vi "CIPT_softwarecontrol probe rework 8 8 23.vi"() -> ()   [LabVIEW 2022 SP3]
uses:
  Git/CIPT/CIPT/Labview Project/CIPT modes.ctl
  <vilib>/Analysis/baseanly.llb/Mean (DBL).vi
  <vilib>/Utility/file.llb/Read Delimited Spreadsheet (DBL).vi
  <vilib>/Utility/file.llb/Read Delimited Spreadsheet (I64).vi
  <vilib>/gmath/NumericalOptimization/Nonlinear Curve Fit LM.vi
  <vilib>/Utility/file.llb/Write Delimited Spreadsheet (string).vi
  <vilib>/Utility/file.llb/Write Delimited Spreadsheet (I64).vi
  <vilib>/Utility/file.llb/Write Delimited Spreadsheet (DBL).vi
  C:/CIPT/Labview Project/Camera Driver/Labview Driver/OtherDrivers/LabVIEW/ueye.NET/uEyeDotNet.dll
  CIPT/Labview Project/Camera Driver/Labview Driver/OtherDrivers/LabVIEW/ueye.NET/uEyeDotNet.dll
  <vilib>/gmath/NI_Gmath.lvlib
  <instrlib>/Keithley DMM6500 DAQ6500 Series/Keithley DMM6500 DAQ6500 Series.lvlib
  <instrlib>/Keithley 24XX/Keithley 24XX.lvlib
  <instrlib>/Keithley 2182/Keithley 2182.lvlib
  <vilib>/Analysis/NI_AALBase.lvlib
panel:
  out "Comms Errors":errorcluster[](array[cluster])
  in  "Save File":bool
  out "error file out":errorcluster
  in  "output file path":path=path "C:/CIPT/Labview Project/csv files/test output.csv"
  in  "stop":bool
  in  "Tab Control":T1(tab)
  in  "Camera ID 3":enum16{"2", "1"}(ring)
  in  "Camera ID 1":enum16{"2", "1"}(ring)
  in  "down a2":bool
  in  "up a2":bool
  in  "down a1":bool
  in  "up a1":bool
  in  "down a3":bool
  in  "up a3":bool
  in  "down all":bool
  in  "up all":bool
  in  "steps /\n continuous \ntoggle":bool
  out "Image first camera":picture
  out "Serial Number 1":string
  in  "Init Camera":bool
  in  "Exit Camera":bool
  in  "Init Camera 2":bool
  in  "Exit Camera 2":bool
  out "Serial Number 2":string
  out "Image second camera":picture
  out "Error Camera 1":errorcluster caption="error"
  out "Error Camera 2":errorcluster caption="error"
  in  "COM 1":refnum<visa-resource-name>
  out "error":errorcluster
  in  "Turn On Landing Test":bool
  in  "Step size":i32=10
  in  "Probe Landing File":path=path "C:/CIPT/Labview Project/csv files/Probe Landing cipt.csv"
  out "Probe List":i64[][](array[numeric])
  out "Resistance":sgl[](array[numeric])
  in  "Probe Threshold (ohm)":dbl
  out "Touching Probes":i64[][](array[numeric])
  out "Loaded":bool
  out "Loaded":bool
  out "Error Probe Configuration File":errorcluster
  in  "Probe Configuration File":path=path "C:/CIPT/Labview Project/csv files/test probe config.csv"
  in  "Probe Settings File":path=path "C:/CIPT/Labview Project/csv files/deafult_probe_setrings.CSV"
  out "Error Probe Settings File":errorcluster
  out "Probe Spacings":dbl[][](array[numeric])
  in  "Load":bool
  in  "Multiplexer":refnum<visa-resource-name>
  out "all rows":i64[][](array[numeric])
  out "Results Description":string[](array[string])
  out "Results":dbl[][](array[numeric])
  out "Probe Set 2":i32
  in  "Compliance voltage (V)":dbl=42.0
  in  "Measure Instrument":refnum<visa-resource-name>
  in  "Radio Buttons":T2 caption="Select Instrumentation"
  in  "Source Instrument":refnum<visa-resource-name>
  in  "Run":bool
  in  "Current (µA)":dbl=10.0
  out "Measurement Log":string
  out "Probe Set":i32
  in  "Measurement Repeats":i32=10
  in  "Size Of Buffer Used For One Measurement":i32=3
  in  "Top Film R est.":dbl=0.25
  in  "Bottm Film R est.":dbl=0.25
  in  "RA est.":dbl=0.25
  out "Top Film R":dbl
  out "Bottom Film R":dbl
  out "RA":dbl
  out "error out (fitting model)":errorcluster
  in  "Fit Data":bool
  out "Measurements Map Out":map{string, dbl[]}(c390)
  # "Probe Landing cipt_probe check: checks probes individually \nProbe Landing cipt: checks for any connection"
  # "All"
  # "End"
  # "home"
  # "Delete"
  # "Insert"
  # "Page Down"
  # "Page up"
  # "F2"
  # "F1"
  # "Steps"
  # "Continuous"
  # "Probe Settings"
  # "Probe Configuration"
  # "I+"
  # "V+"
  # "V-"
  # "I-"
  # "Max Resolution of 2400 is 300 µV in 200 mV range"
  # "/"
  # "Sheet Resistance (RA)"
  # "Estimated Values"
  # "Fitted Values"
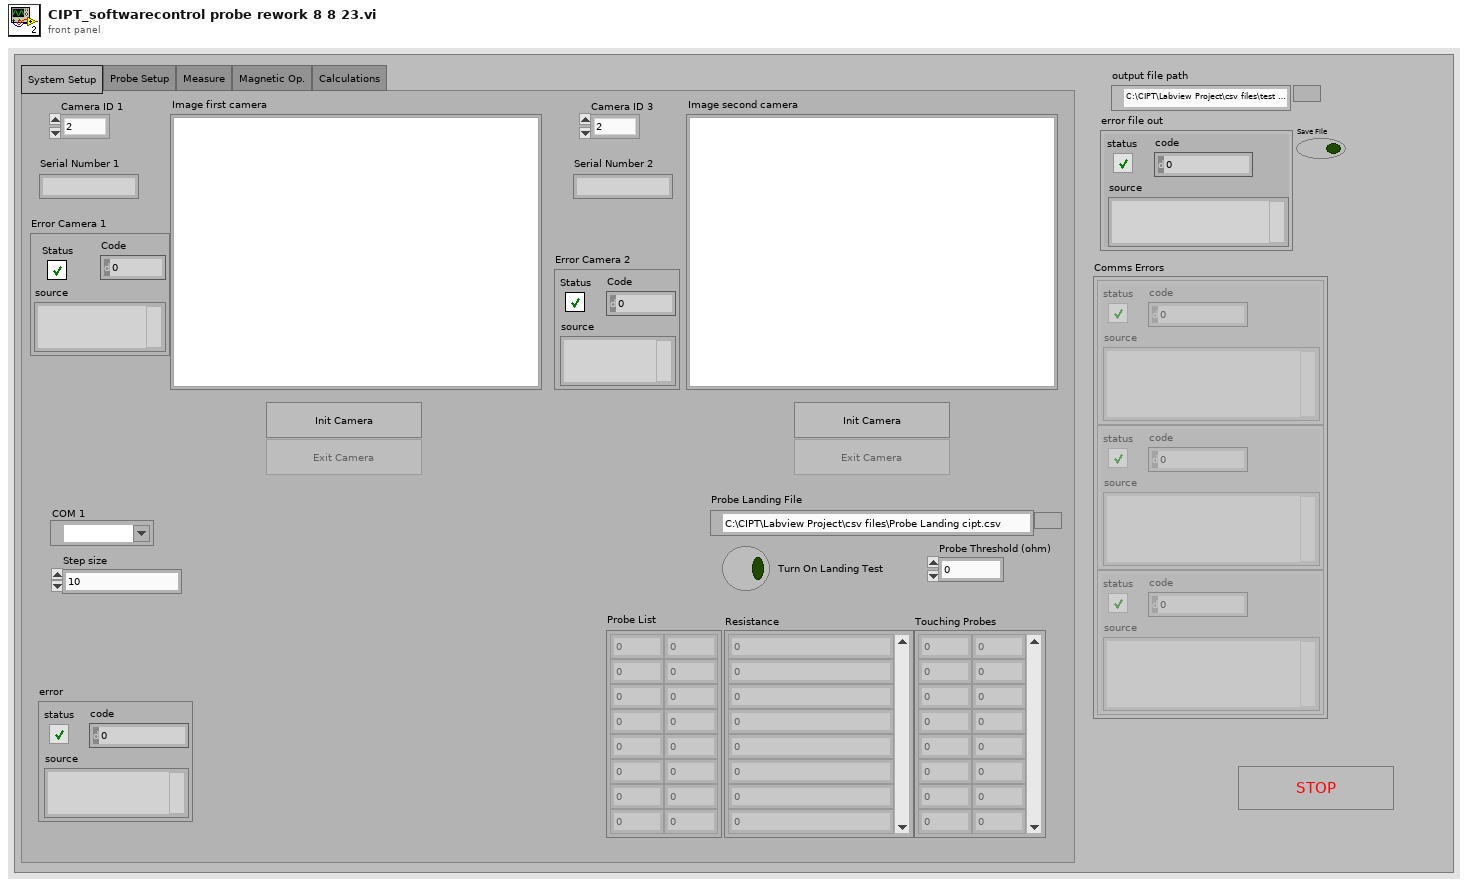
[diagram p1: front panel]
types:
  T1 = enum32{"System Setup", "Probe Setup", "Measure", "Magnetic Op.", "Calculations"}
  T2 = typedef "CIPT modes.ctl" = enum32{"DAQ6510", "2400 Only", "2400 and  2182", "SR830", "SR830 and 6221"}
  T3 = enum32{"System Setup", "Probe Setup", "Measure", "Magnetic Operations", "Calculations + Analyis"}
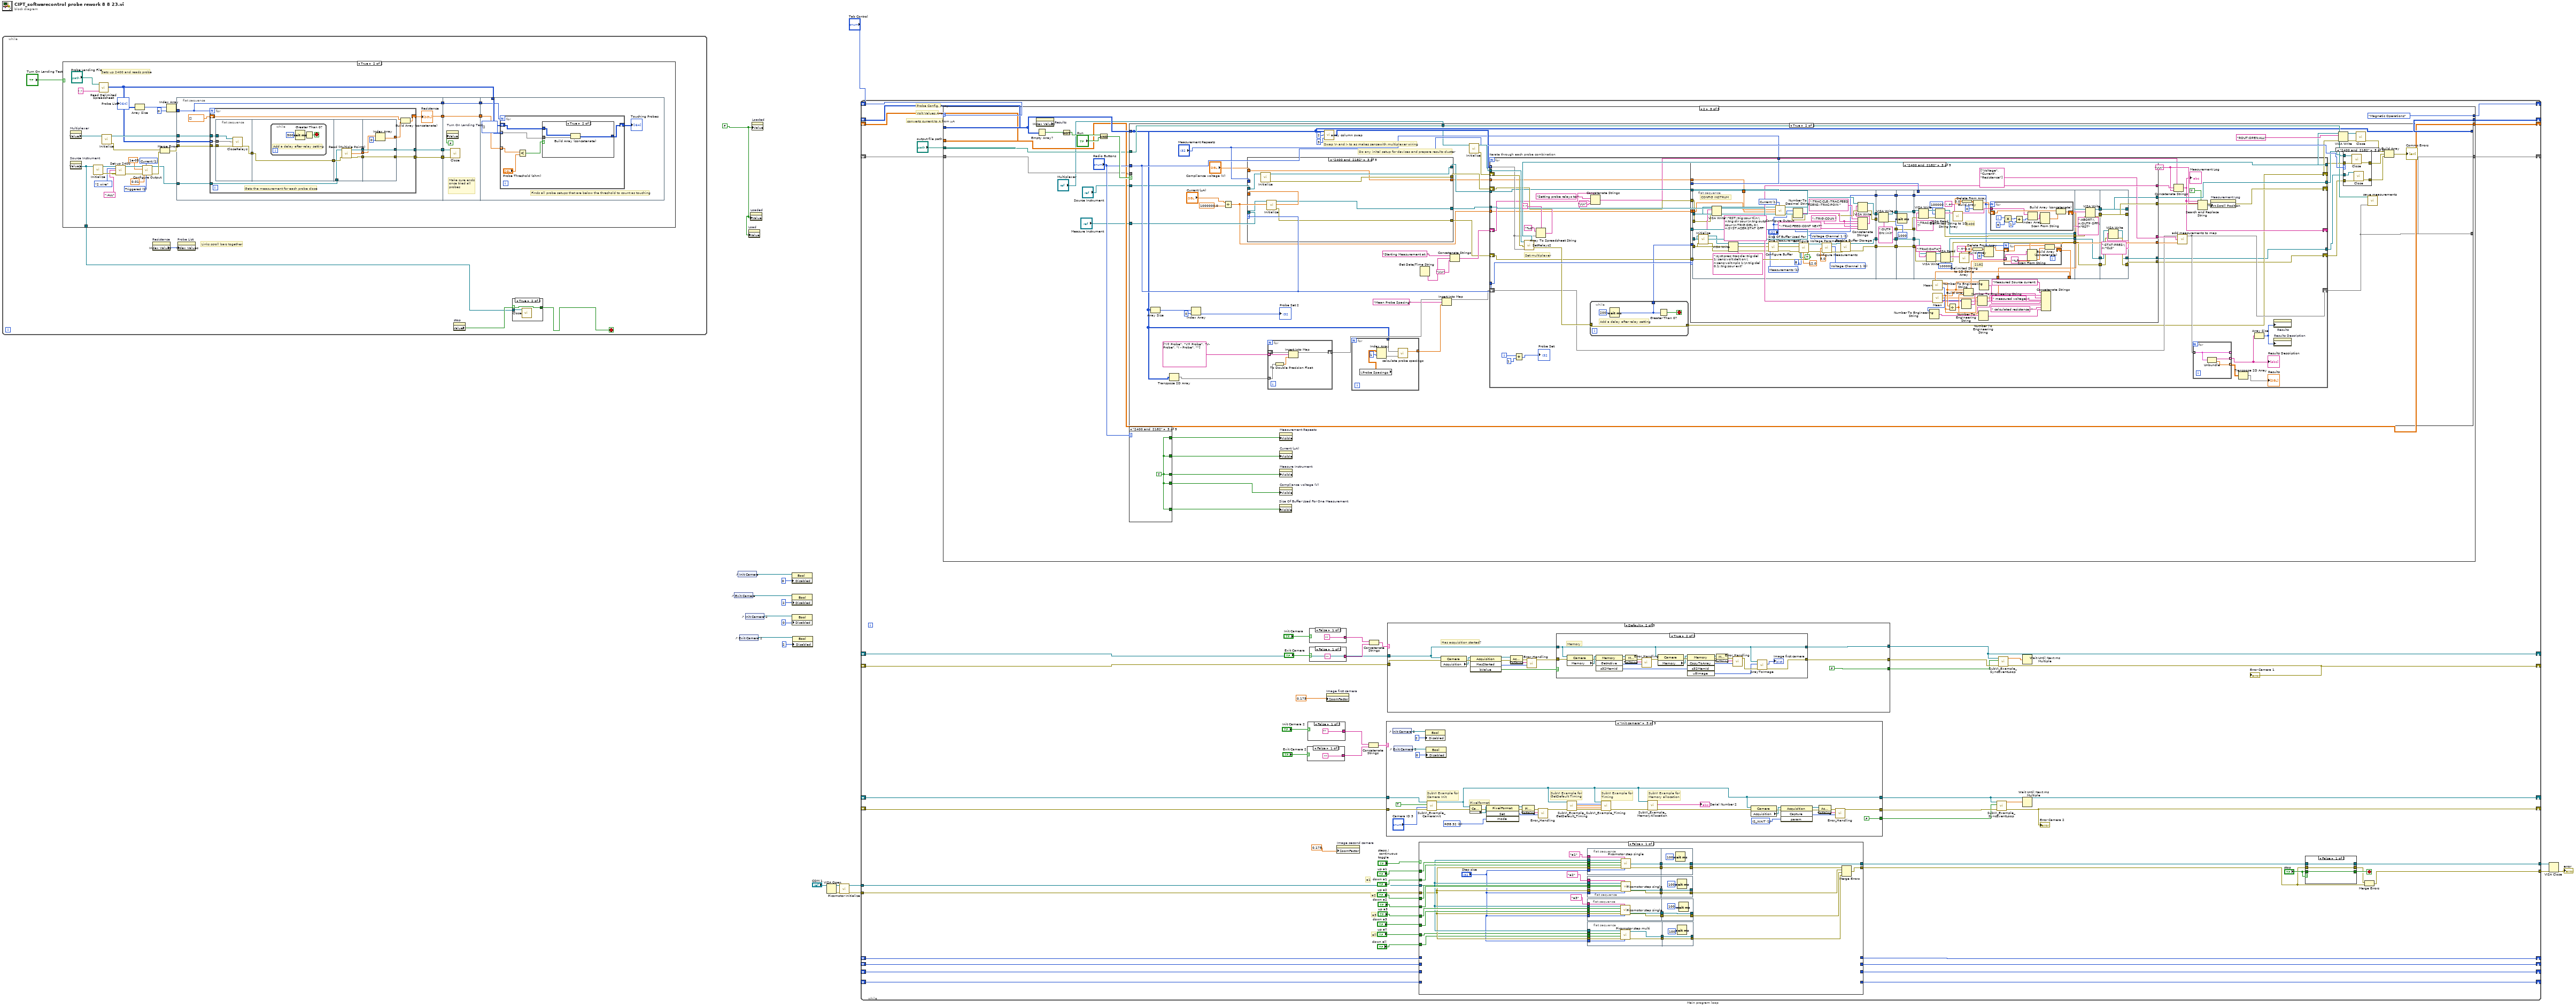
[diagram p0: block diagram]
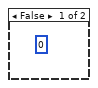
[diagram p3: hidden frame]
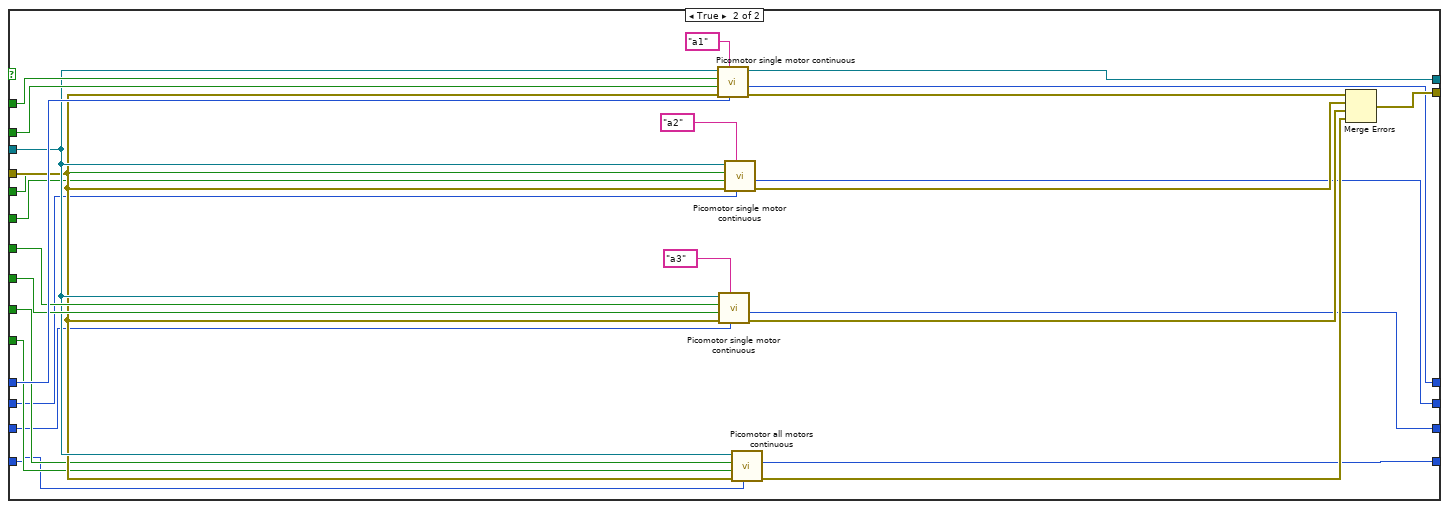
[diagram p5: hidden frame]
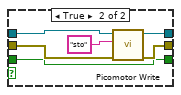
[diagram p6: hidden frame]
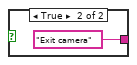
[diagram p7: hidden frame]
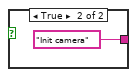
[diagram p8: hidden frame]
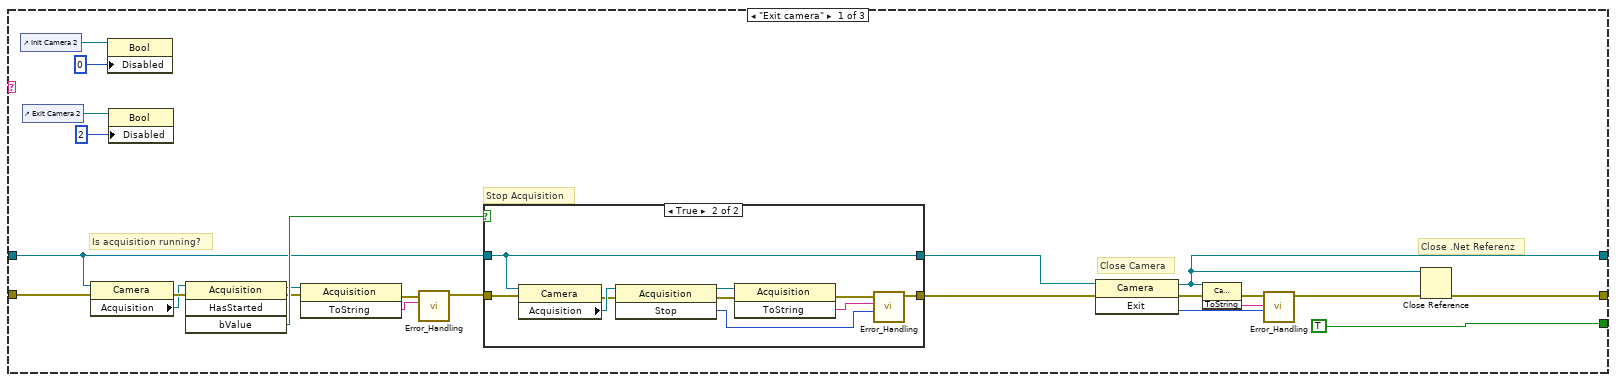
[diagram p9: hidden frame]
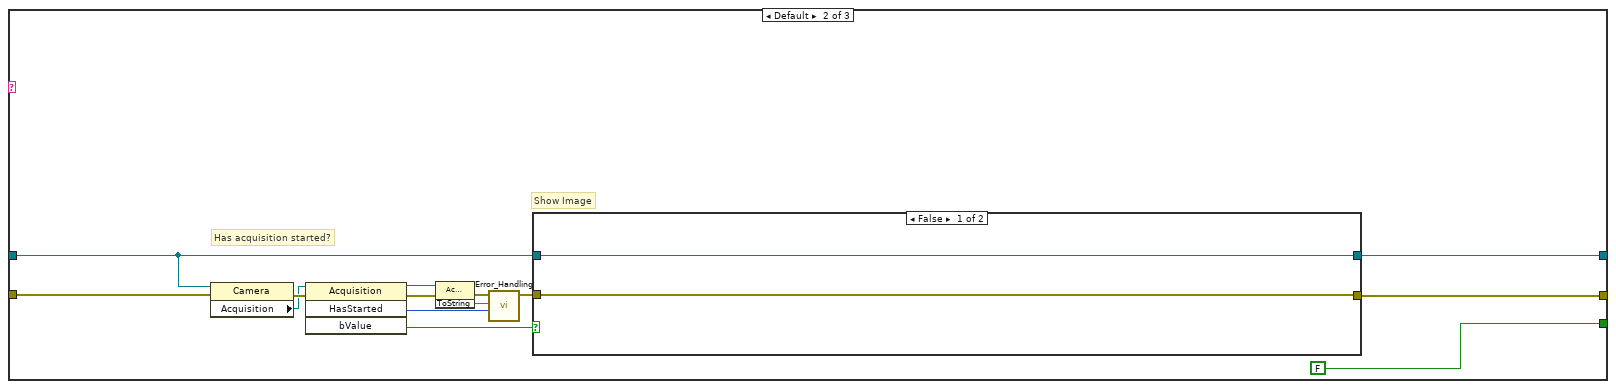
[diagram p11: hidden frame]
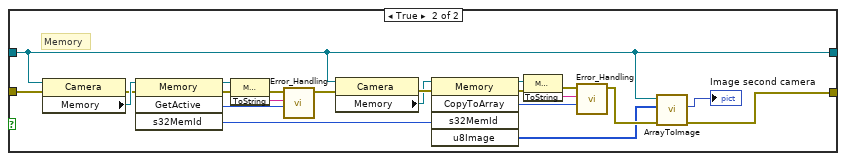
[diagram p12: hidden frame]
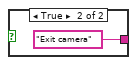
[diagram p13: hidden frame]
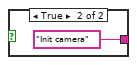
[diagram p14: hidden frame]
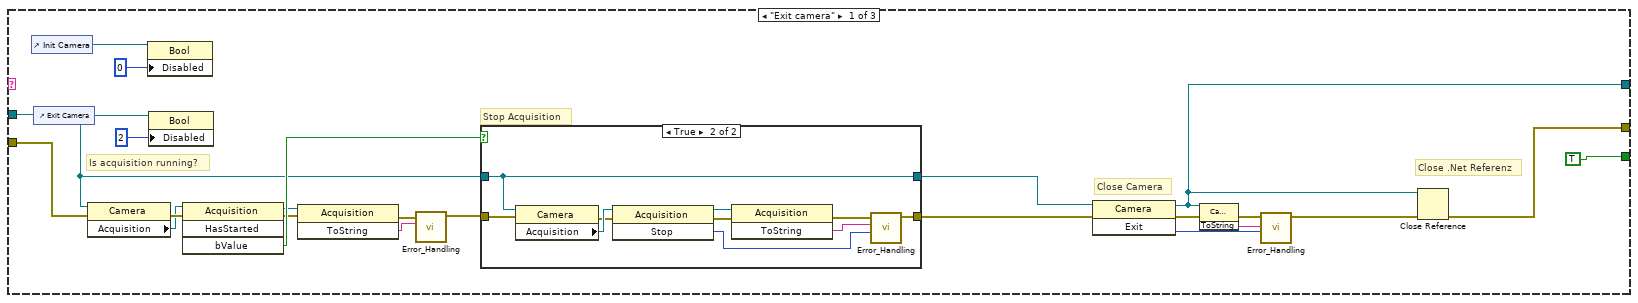
[diagram p15: hidden frame]
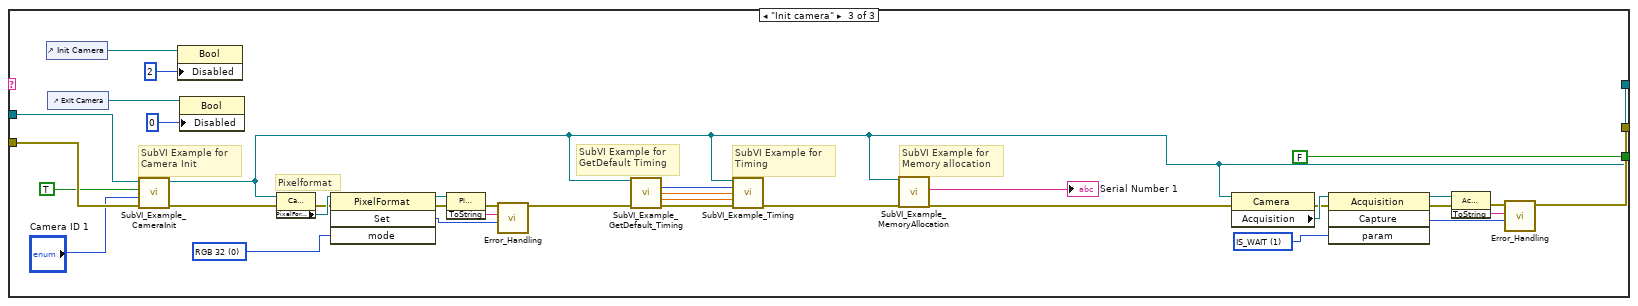
[diagram p18: hidden frame]
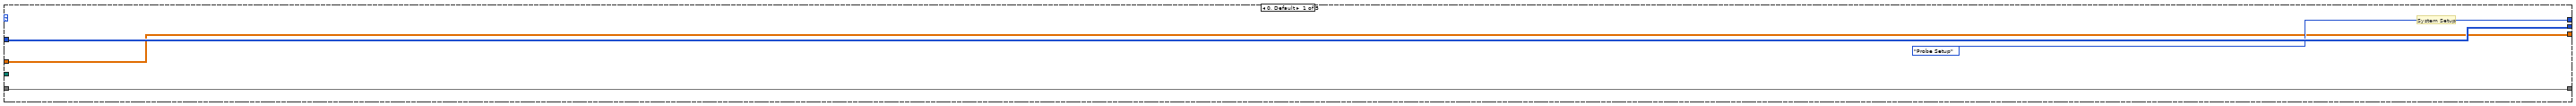
[diagram p19: hidden frame]
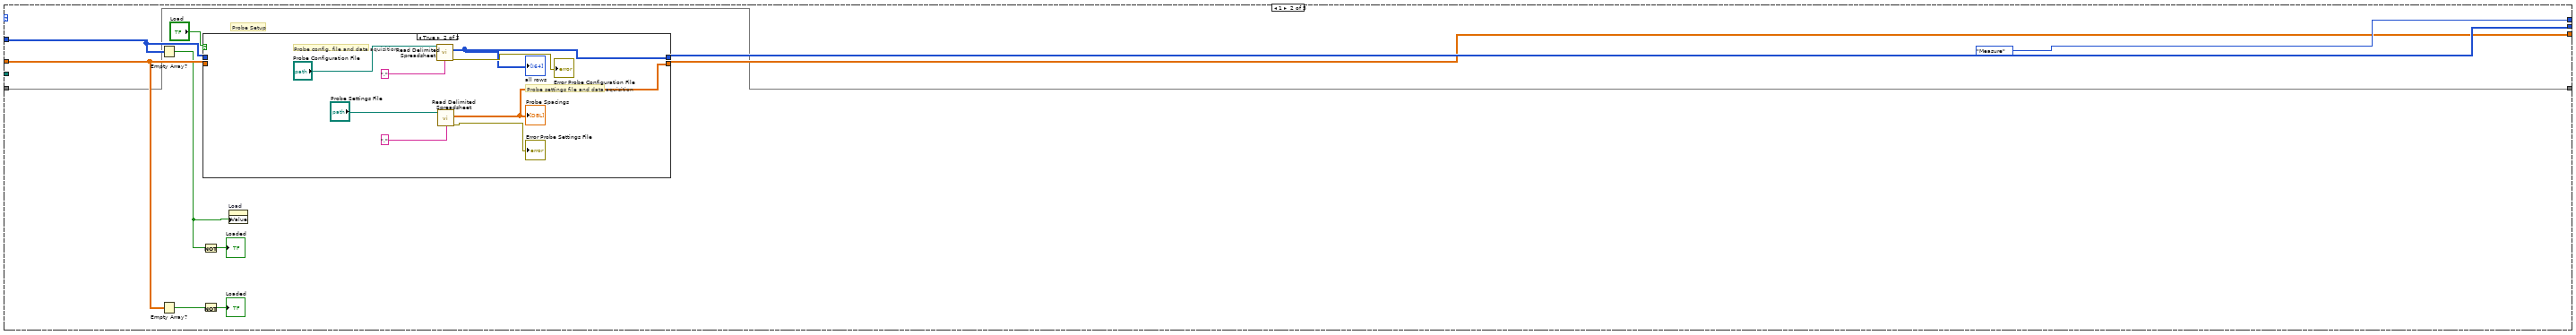
[diagram p20: hidden frame]
diagram:
  w9 = FALSE
  n1 = while {
    stop <- w23 stop-if-true
    # "Links scroll bars together"
    n2 = case shown="True" "Turn On Landing Test" {
      tunnel: [_ w32] -> w20
      frame False {
        (unwired) 0
      }
      frame True {
        w49 = u16 1 items=["Immediate", "Triggered"] ("Output Type  (0: Immediate)")
        w48 = u16 1 items=["Voltage", "Current"] ("Source Mode  (0: Voltage)")
        # "Sets up 2400 and reads probe"
        n3 = property on="Multiplexer" class="VISAName"() -> ("Value"=w43:refnum<visa-resource-name>)  [unwired: 2 in, 2 out]
        n4 = property on="Source Instrument" class="VISAName"() -> ("Value"=w32:refnum<visa-resource-name>)  [unwired: 2 in, 2 out]
        n5 = call <instrlib>:"Initialize.vi"("VISA resource name"=w32) -> ("error out"=w51:errorcluster, "VISA resource name out"=w50:refnum<visa-resource-name>)  [unwired: 9 in]
        n6 = call-poly <vilib>:"Read Delimited Spreadsheet.vi"("file path (dialog if empty)"="Probe Landing File", "delimiter (\\t)"="," ("delimiter (\\t)")) -> ("all rows"=w29:i64[][])  [unwired: 8 in, 5 out]
        "Probe List" <- w29
        n7 = call <instrlib>:"Initialize.vi"("VISA resource name"=w43) -> ("error out"=w41:errorcluster, "VISA resource name out"=w36:refnum<visa-resource-name>)  [unwired: 9 in]
        n8 = call "Set up 2400.vi"("VISA resource name"=w50, "Sense mode"=enum16{"2 wire", "4 wire"}."2 wire", "Measurement Function"=":ALL", "error in (no error)"=w51) -> ("VISA resource name out"=w52:refnum<visa-resource-name>, "error out"=w53:errorcluster)  [unwired: 10 in]
        n9 = Array Size(array=w29) -> (size(s)=w40:i32[])
        n10 = call <instrlib>:"Configure Output.vi"("Output Type  (0: Immediate)"=w49, "Source Mode  (0: Voltage)"=w48, "error in (no error)"=w53, "Compliance  Level (0.1)"=0.01, "Output Level (0)"=1e-05, "VISA resource name"=w52) -> ("error out"=w42:errorcluster, "VISA resource name out"=w35:refnum<visa-resource-name>)  [unwired: 4 in]
        n11 = Merge Errors(w41, w42) -> (w37:errorcluster)
        n12 = Index Array(array=w40, index=0) -> (element=w38:i32)
        n13 = flat-sequence {
          tunnel: w38 -> [w57]
          tunnel: w37 -> [w64]
          tunnel: w36 -> [w63]
          tunnel: w29 -> [w62]
          tunnel: w35 -> [w61]
          tunnel: [w60] -> w34
          tunnel: [w59] -> w33
          tunnel: [w58] -> w30
          tunnel: [w57] -> w27
          tunnel: w34 -> [w100]
          tunnel: w33 -> [w99]
          tunnel: [w98] -> w31
          tunnel: w30 -> [w98]
          tunnel: [w97] -> w28
          tunnel: w27 -> [w97]
          tunnel: w31 -> [w106]
          tunnel: w29 -> [w105]
          tunnel: w28 -> [w104]
          frame #0 {
            n14 = for {
              N: w57 -> [_]
              tunnel: w64 -> [w76]
              tunnel: w63 -> [w75]
              tunnel: w62 -> [w74] mode=indexing
              shift-right: [w69] -> w58
              shift-left: dbl[] [] -> [w68]
              tunnel: w61 -> [w67]
              tunnel: [w66] -> w60
              tunnel: [w65] -> w59
              # "Gets the measurement for each probe close"
              n15 = flat-sequence {
                tunnel: [w82] -> w78
                tunnel: w76 -> [w81]
                tunnel: w75 -> [w80]
                tunnel: w74 -> [w79]
                tunnel: [w83] -> w77
                tunnel: w78 -> [w83]
                tunnel: w77 -> [w91]
                tunnel: [w90] -> w73
                tunnel: [w89] -> w72
                tunnel: [w88] -> w71
                tunnel: w67 -> [w87]
                tunnel: [w95] -> w65
                tunnel: [w96] -> w66
                tunnel: w73 -> [w96]
                tunnel: w72 -> [w95]
                tunnel: w71 -> [w93]
                tunnel: [w92] -> w70
                frame #0 {
                  n16 = call "CloseRelays.vi"("error in (no error)"=w81, "Array"=w79, "VISA Refnum in"=w80) -> ("error out"=w82:errorcluster)  [unwired: 6 in, 2 out]
                }
                frame #1 {
                  n17 = while {
                    stop <- w85 stop-if-true
                    # "Add a delay after relay setting"
                    n18 = Wait (ms)(milliseconds to wait=u32 500) -> (millisecond timer value=w84:u32)
                    n19 = Greater Than 0?(x=w84) -> (x > 0?=w85:bool)
                  }
                }
                frame #2 {
                  n20 = call <instrlib>:"Read (Multiple Points).vi"("VISA resource name"=w87, "error in (no error)"=w91) -> ("VISA resource name out"=w90:refnum<visa-resource-name>, "Resistance"=w88:sgl[], "error out"=w89:errorcluster)  [unwired: 7 in, 4 out]
                }
                frame #3 {
                  n21 = Index Array(array=w93, index=0) -> (element=w92:sgl)
                }
              }
              n22 = Build Array (concatenate)(w68, w70) -> (w69:dbl[])
            }
            "Resistance" <- w58
          }
          frame #1 {
            # "Make sure ends once tried all probes"
            n23 = property on="Turn On Landing Test" class="Bool (strict)"("Value"=FALSE) -> ()  [unwired: 2 in, 2 out]
            n24 = call <instrlib>:"Close.vi"("error in (no error)"=w99, "VISA resource name"=w100) -> ()  [unwired: 9 in, 1 out]
          }
          frame #2 {
            # "Finds all probe setups that are below the threshold to count as touching"
            n25 = for {
              N: w104 -> [_]
              tunnel: w106 -> [w111] mode=indexing
              tunnel: w105 -> [w109] mode=indexing
              shift-right: [w108] -> w103
              shift-left: i64[][] [] -> [w107]
              n26 = Less?(x=w111, y="Probe Threshold (ohm)") -> (x < y?=w110:bool)
              n27 = case shown="True" w110 {
                tunnel: w109 -> [_ w116]
                tunnel: [w113 w115] -> w108
                tunnel: w107 -> [w113 w114]
                frame False {
                }
                frame True {
                  n28 = Build Array (concatenate)(w114, w116) -> (w115:i64[][])
                }
              }
            }
            "Touching Probes" <- w103
          }
        }
      }
    }
    n29 = property on="Resistance" class="Arr (strict)"() -> ("Index Values"=w19:u32[])  [unwired: 2 in, 2 out]
    n30 = property on="Probe List" class="Arr (strict)"("Index Values"=w19) -> ()  [unwired: 2 in, 2 out]
    n31 = property on="stop" class="Bool (strict)"() -> ("Value"=w21:bool)  [unwired: 2 in, 2 out]
    n32 = case shown="True" w21 {
      selector: w21 -> [w24 w26]
      tunnel: [w24 w26] -> w23
      tunnel: w20 -> [_ w25]
      frame False {
      }
      frame True {
        n33 = call <instrlib>:"Close.vi"("VISA resource name"=w25) -> ()  [unwired: 10 in, 1 out]
      }
    }
  }
  n34 = control-ref of="Exit Camera"() -> (w12:refnum<vi>)
  n35 = control-ref of="Init Camera"() -> (w13:refnum<vi>)
  n36 = control-ref of="Exit Camera 2"() -> (w17:refnum<vi>)
  n37 = control-ref of="Init Camera 2"() -> (w16:refnum<vi>)
  n38 = property on="Load" class="Bool (strict)"("Value"=w9) -> ()  [unwired: 2 in, 2 out]
  n39 = property on="Loaded" class="Bool (strict)"("Value"=w9) -> ()  [unwired: 2 in, 2 out]
  n40 = property on="Loaded" class="Bool (strict)"("Value"=w9) -> ()  [unwired: 2 in, 2 out]
  n41 = property class="Bool"(reference=w13, "Disabled"=u8 0 ("Deaktiviert")) -> ()  [unwired: 1 in, 2 out]
  n42 = property class="Bool"(reference=w12, "Disabled"=u8 2 ("Deaktiviert")) -> ()  [unwired: 1 in, 2 out]
  n43 = property class="Bool"(reference=w16, "Disabled"=u8 0 ("Deaktiviert")) -> ()  [unwired: 1 in, 2 out]
  n44 = property class="Bool"(reference=w17, "Disabled"=u8 2 ("Deaktiviert")) -> ()  [unwired: 1 in, 2 out]
  n45 = VISA Open(VISA resource name="COM 1") -> (VISA resource name=w7:refnum<visa-resource-name>, error out=w6:errorcluster)  [unwired: 4 in]
  n46 = call "Picomotor Initialize.vi"("error in (no error)"=w6, "VISA Refnum in"=w7) -> ("error out"=w4:errorcluster, "VISA Refnum out"=w5:refnum<visa-resource-name>)  [unwired: 8 in]
  n47 = while "Main program loop" {
    shift-right: [w175] -> _
    shift-left: _ -> [w176]
    shift-right: [w174] -> _
    shift-left: "Tab Control" -> [w177]
    shift-right: [w173] -> _
    shift-left: _ -> [w172]
    shift-right: [w170] -> _
    shift-left: _ -> [w169]
    shift-right: [w158] -> _
    shift-left: _ -> [w156]
    shift-right: [w159] -> _
    shift-left: _ -> [w157]
    shift-right: [w146] -> _
    shift-left: _ -> [w144]
    shift-right: [w145] -> _
    shift-left: _ -> [w143]
    tunnel: w5 -> [w130]
    tunnel: w4 -> [w129]
    tunnel: [w142] -> w2
    shift-right: [w127] -> _
    shift-left: _ -> [w123]
    shift-right: [w126] -> _
    shift-left: _ -> [w122]
    shift-right: [w125] -> _
    shift-left: _ -> [w121]
    shift-right: [w124] -> _
    shift-left: _ -> [w120]
    tunnel: [w117] -> w1
    stop <- w141 stop-if-true
    # "a2"
    # "a3"
    # "all"
    # "a1"
    # "converts current to A from µA"
    # "Volt Values Array"
    # "Probe Config. Array"
    n48 = case shown="2" w177 {
      tunnel: w176 -> [w516 w523 w553 w912 w919]
      tunnel: [w516 w527 w552 w912 w919] -> w175
      tunnel: [T3."Probe Setup" ("Tab Control") T3."Measure" ("Tab Control") T3."Magnetic Operations" ("Tab Control") T3."Calculations + Analyis" ("Tab Control") T3."System Setup" ("Tab Control")] -> w174
      tunnel: [w514 w522 w547 w911 w918] -> w173
      tunnel: w172 -> [w514 w521 w547 w911 w918]
      tunnel: "output file path" -> [_ _ w544 _ w917]
      tunnel: [w513 w518 w543 w910 w916] -> w170
      tunnel: w169 -> [w513 w518 w542 w910 w916]
      frame 0, Default {
        # "System Setup"
      }
      frame 1 {
        # "Probe Setup"
        n49 = Empty Array?(array=w523) -> (empty?=w517:bool)
        n50 = Empty Array?(array=w521) -> (empty?=w520:bool)
        n51 = Not(x=w517) -> (.not. x?=→"Loaded":bool)
        n52 = Not(x=w520) -> (.not. x?=→"Loaded":bool)
        n53 = case shown="True" "Load" {
          tunnel: [w529 w530] -> w527
          tunnel: w523 -> [w529 _]
          tunnel: [w528 w531] -> w522
          tunnel: w521 -> [w528 _]
          frame False {
          }
          frame True {
            # "Probe config. file and data aquisition"
            # "Probe settings file and data aquisition"
            n54 = call-poly <vilib>:"Read Delimited Spreadsheet.vi"("file path (dialog if empty)"="Probe Configuration File", "delimiter (\\t)"="," ("delimiter (\\t)")) -> ("all rows"=w530:i64[][], "error out"=→"Error Probe Configuration File":errorcluster)  [unwired: 8 in, 4 out]
            "all rows" <- w530
            n55 = call-poly <vilib>:"Read Delimited Spreadsheet.vi"("file path (dialog if empty)"="Probe Settings File", "delimiter (\\t)"="," ("delimiter (\\t)")) -> ("all rows"=w531:dbl[][], "error out"=→"Error Probe Settings File":errorcluster)  [unwired: 8 in, 4 out]
            "Probe Spacings" <- w531
          }
        }
        n56 = property on="Load" class="Bool (strict)"("Value"=w517) -> ()  [unwired: 2 in, 2 out]
      }
      frame 2 {
        n57 = property on="Results" class="Arr (strict)" props=["Index Values"]() -> ()  [unwired: 2 in, 3 out]
        n58 = Empty Array?(array=w553) -> (empty?=w555:bool)
        n59 = Not(x=w555) -> (.not. x?=w554:bool)
        n60 = Compound Arithmetic op=AND(w554, "Run") -> (w557:bool)
        n61 = case shown="True" w557 {
          tunnel: w553 -> [w568 w587]
          tunnel: [w568 w587] -> w552
          tunnel: "Radio Buttons" -> [_ w613]
          tunnel: w544 -> [_ w601]
          tunnel: [w567 w583] -> w543
          tunnel: w542 -> [w567 _]
          tunnel: "Measure Instrument" -> [_ w575]
          tunnel: "Source Instrument" -> [_ w574]
          tunnel: "Multiplexer" -> [_ w573]
          frame False {
          }
          frame True {
            # "Swap V- and I- to as makes sensewith multiplexer wiring"
            # "Do any inital setup for devices and prepare results cluster"
            n62 = Array Size(array=w587) -> (size(s)=w607:i32[])
            n63 = Transpose 2D Array(2D array=w587) -> (transposed array=w586:i64[][])
            n64 = Index Array "Index Array"(array=w607, index=0) -> (element=→"Probe Set 2":i32)
            n65 = Divide(x="Current (µA)", y=1000000.0) -> (x/y=w569:dbl)
            n66 = case shown="\"2400 and  2182\"" w613 {
              tunnel: w574 -> [_ w651 w657 _ _]
              tunnel: [_ w639 w656 _ _] -> w614
              tunnel: w575 -> [_ _ w658 _ _]
              tunnel: [_ w639 w654 _ _] -> w577
              tunnel: [_ w645 w653 _ _] -> w608
              tunnel: w569 -> [_ w642 _ _ _]
              tunnel: "Compliance voltage (V)" -> [_ w640 w652 _ _]
              tunnel: "Measurement Repeats" -> [_ _ _ _ _]
              tunnel: [_ _ w655 _ _] -> w572
              tunnel: [_ _ w652 _ _] -> w570
              frame "DAQ6510", Default {
              }
              frame "2400 Only" {
                w643 = u16 1 items=["Immediate", "Triggered"] ("Output Type  (0: Immediate)")
                w644 = u16 1 items=["Voltage", "Current"] ("Source Mode  (0: Voltage)")
                n67 = call <instrlib>:"Initialize.vi"("VISA resource name"=w651) -> ("error out"=w649:errorcluster, "VISA resource name out"=w650:refnum<visa-resource-name>)  [unwired: 9 in]
                n68 = call "Set up 2400.vi"("VISA resource name"=w650, "Sense mode"=enum16{"2 wire", "4 wire"}."4 wire", "Measurement Function"=":ALL", "error in (no error)"=w649) -> ("VISA resource name out"=w647:refnum<visa-resource-name>, "error out"=w646:errorcluster)  [unwired: 10 in]
                n69 = call <instrlib>:"Configure Output.vi"("Output Type  (0: Immediate)"=w643, "Source Mode  (0: Voltage)"=w644, "error in (no error)"=w646, "Compliance  Level (0.1)"=w640, "Output Level (0)"=w642, "VISA resource name"=w647) -> ("error out"=w645:errorcluster, "VISA resource name out"=w639:refnum<visa-resource-name>)  [unwired: 4 in]
              }
              frame "2400 and  2182" {
                n70 = call <instrlib>:"Initialize.vi"("VISA resource name"=w657) -> ("error out"=w653:errorcluster, "VISA resource name out"=w654:refnum<visa-resource-name>)  [unwired: 9 in]
                n71 = call <instrlib>:"Initialize.vi"("VISA resource name"=w658) -> ("error out"=w655:errorcluster, "VISA resource name out"=w656:refnum<visa-resource-name>)  [unwired: 9 in]
              }
              frame "SR830" {
              }
              frame "SR830 and 6221" {
              }
            }
            n72 = for {
              tunnel: w586 -> [w625] mode=indexing
              tunnel: string[] ["I+ Probe", "V+ Probe", "V- Probe", "I - Probe", ""] -> [w626] mode=indexing
              shift-right: [w623] -> w591
              shift-left: _ -> [w622]
              n73 = To Double Precision Float(number=w625) -> (double precision float=w624:dbl[])
              n74 = Insert Into Map(map in=w622, key=w626, value=w624) -> (map out=w623:map{string, dbl[]})  [unwired: 2 out]
            }
            n75 = call "array column swap.vi"("Collumn 2 index"=3, "Collumn 1 index"=2, "Input array"=w587) -> ("output array"=w604:i32[][])
            n76 = for {
              tunnel: w587 -> [w618] mode=indexing
              tunnel: [w617] -> w590 mode=indexing
              n77 = local read "Probe Spacings"() -> (w621:dbl[][])
              n78 = Index Array(array=w621, index (row)=1) -> (element=w619:dbl[])  [unwired: 1 in]
              n79 = call "calculate probe spacings.vi"("Probe Spacings"=w619, "Probe list"=w618) -> ("Mean Spacing"=w617:dbl)  [unwired: 1 out]
            }
            n80 = Get Date/Time String() -> (time string=w610:string)  [unwired: 3 in, 1 out]
            n81 = Insert Into Map(map in=w591, key="Mean Probe Spacing", value=w590) -> (map out=w588:map{string, dbl[]})  [unwired: 2 out]
            n82 = Concatenate Strings("Starting Measurement at: ", w610, "\r\n") -> (w599:string)
            n83 = call <instrlib>:"Initialize.vi"("VISA resource name"=w573) -> ("error out"=w615:errorcluster, "VISA resource name out"=w616:refnum<visa-resource-name>)  [unwired: 9 in]
            n84 = for "Iterate through each probe combination" {
              tunnel: w616 -> [w700]
              tunnel: [w699] -> w597
              tunnel: w604 -> [w693] mode=indexing
              tunnel: w613 -> [w698]
              tunnel: w614 -> [w696]
              shift-right: [w682] -> _
              shift-left: w599 -> [w683]
              shift-right: [w694] -> w611
              shift-left: w608 -> [w687]
              shift-right: [w673] -> w583
              shift-left: w588 -> [w675]
              shift-right: [w667] -> w584
              shift-left: w572 -> [w668]
              tunnel: w577 -> [w686]
              tunnel: [w695] -> w612
              shift-right: [w670] -> w579
              shift-left: w615 -> [w697]
              tunnel: [w666] -> w585
              tunnel: "Measurement Repeats" -> [w665]
              tunnel: w570 -> [w661]
              tunnel: w569 -> [w660]
              i -> [w664]
              w680 = "\r\n"
              # "Set multiplexer"
              n85 = Add(x=w664, y=1) -> (x+y=→"Probe Set":i32)
              n86 = call "SetRelays2.vi"("all rows"=w693, "error in (no error)"=w697, "VISA Refnum in"=w700) -> ("error out"=w688:errorcluster, "VISA resource name out"=w699:refnum<visa-resource-name>)  [unwired: 1 in]
              n87 = Array To Spreadsheet String(delimiter (Tab)=",", array=w693, 3:"%d" ("format string")) -> (spreadsheet string=w689:string)
              n88 = while {
                tunnel: [w707] -> w670
                tunnel: w688 -> [w707]
                tunnel: [w704] -> w669
                stop <- w705 stop-if-true
                # "Add a delay after relay setting"
                n89 = Wait (ms)(milliseconds to wait=u32 200) -> (millisecond timer value=w704:u32)
                n90 = Greater Than 0?(x=w704) -> (x > 0?=w705:bool)
              }
              n91 = Concatenate Strings(w683, "Setting probe relays to:", w689, "\r\n") -> (w678:string)
              n92 = case shown="\"2400 and  2182\"" w698 {
                tunnel: w696 -> [w709 w713 w778 w902 w906]
                tunnel: w686 -> [w708 w734 w786 w903 w907]
                tunnel: w687 -> [w710 w733 w785 w904 w908]
                tunnel: [w708 w731 w746 w903 w907] -> w695
                tunnel: [w710 w730 w754 w904 w908] -> w694
                tunnel: [_ w723 w779 _ _] -> w684
                tunnel: w665 -> [_ w722 w784 _ _]
                tunnel: [_ w716 w783 _ _] -> w676
                tunnel: [_ string[] ["Voltage", "Current", "Resistance"] string[] ["Voltage", "Current", "Resistance"] _ _] -> w677
                tunnel: w669 -> [_ _ _ _ _]
                tunnel: w668 -> [w711 w714 w777 w905 w909]
                tunnel: [w711 w714 w750 w905 w909] -> w667
                tunnel: [w709 w713 w747 w902 w906] -> w666
                tunnel: w661 -> [_ _ w739 _ _]
                tunnel: w660 -> [_ _ w738 _ _]
                frame "DAQ6510", Default {
                }
                frame "2400 Only" {
                  w732 = u16 0 items=["Fixed", "Sweep", "List"] ("Output Mode (0: Fixed)")
                  n93 = call <instrlib>:"Read (Multiple Points).vi"("VISA resource name"=w734, "Sample Count (1)"=w722, "error in (no error)"=w733, "Output Mode (0: Fixed)"=w732) -> ("Voltage"=w712:sgl[], "VISA resource name out"=w731:refnum<visa-resource-name>, "Current"=w721:sgl[], "Resistance"=w720:sgl[], "error out"=w730:errorcluster)  [unwired: 5 in, 2 out]
                  n94 = call-poly <vilib>:"Mean.vi"("X"=w712) -> ("mean"=w719:dbl)  [unwired: 1 out]
                  n95 = call-poly <vilib>:"Mean.vi"("X"=w721) -> ("mean"=w718:dbl)  [unwired: 1 out]
                  n96 = call-poly <vilib>:"Mean.vi"("X"=w720) -> ("mean"=w717:dbl)  [unwired: 1 out]
                  n97 = Build Array(w719, w718, w717) -> (w716:dbl[])
                  n98 = Number To Engineering String(4:w719) -> (0:w724:string)  [unwired: 3 in]
                  n99 = Number To Engineering String(4:w718) -> (0:w728:string)  [unwired: 3 in]
                  n100 = Number To Engineering String(4:w717) -> (0:w725:string)  [unwired: 3 in]
                  n101 = Concatenate Strings("Measured I = ", w728, " V = " ("string"), w724, "R = " ("string"), w725) -> (w723:string)
                }
                frame "2400 and  2182" {
                  n102 = flat-sequence {
                    tunnel: w777 -> [w793]
                    tunnel: w778 -> [w794]
                    tunnel: w785 -> [w795]
                    tunnel: w786 -> [w796]
                    tunnel: [w800] -> w749
                    tunnel: [w799] -> w748
                    tunnel: [w798] -> w741
                    tunnel: [w797] -> w740
                    tunnel: w739 -> [w791]
                    tunnel: w738 -> [w790]
                    tunnel: ["Size Of Buffer Used For One Measurement"] -> w735
                    tunnel: [w833] -> w766
                    tunnel: [w832] -> w764
                    tunnel: [w830] -> w761
                    tunnel: [w829] -> w759
                    tunnel: w749 -> [w833]
                    tunnel: w748 -> [w832]
                    tunnel: w741 -> [w831]
                    tunnel: w740 -> [_]
                    tunnel: [w827] -> w736
                    tunnel: w735 -> [w827]
                    tunnel: w766 -> [w839]
                    tunnel: [w839] -> w765
                    tunnel: w764 -> [w838]
                    tunnel: [w838] -> w763
                    tunnel: [w836] -> w762
                    tunnel: w761 -> [w836]
                    tunnel: [w835] -> w760
                    tunnel: w759 -> [w835]
                    tunnel: [w834] -> w737
                    tunnel: w736 -> [w834]
                    tunnel: w784 -> [_]
                    tunnel: w765 -> [w849]
                    tunnel: w763 -> [w848]
                    tunnel: w762 -> [w851]
                    tunnel: w760 -> [w850]
                    tunnel: [w847] -> w758
                    tunnel: [w846] -> w757
                    tunnel: [w844] -> w756
                    tunnel: [w843] -> w755
                    tunnel: [w842] -> w752
                    tunnel: [w841] -> w751
                    tunnel: w737 -> [w840]
                    tunnel: w756 -> [w894]
                    tunnel: w755 -> [w893]
                    tunnel: w752 -> [w889]
                    tunnel: w751 -> [w890]
                    tunnel: [w891] -> w745
                    tunnel: [w890] -> w744
                    tunnel: [w889] -> w743
                    tunnel: [w888] -> w742
                    tunnel: [w900] -> w746
                    tunnel: [w895] -> w747
                    tunnel: [w896] -> w750
                    tunnel: [w901] -> w754
                    tunnel: w745 -> [w901]
                    tunnel: w744 -> [w897]
                    tunnel: w743 -> [w898]
                    tunnel: w742 -> [w900]
                    frame #0 {
                      w804 = 0 items=["Voltage Channel 1", "Voltage Channel 2", "Temperature Channel 1", "Temperature Channel 2"] ("Measurement (0: Voltage Channel 1)")
                      w792 = u16 1 items=["Voltage", "Current"] ("Source Mode  (0: Voltage)")
                      w817 = 1 items=["Voltage Channel 1"=1, "Voltage Channel 2"=2] ("Measurement (1: Voltage Channel 1)")
                      w818 = 1 items=["None", "Measurements", "Math Calculation"] ("Buffer Source (0: None)")
                      # "CONFIG INSTRUM"
                      n103 = call <instrlib>:"Initialize.vi"("error in (no error)"=w793, "VISA resource name"=w794) -> ("error out"=w802:errorcluster, "VISA resource name out"=w803:refnum<visa-resource-name>)  [unwired: 8 in]
                      n104 = VISA Write(VISA resource name=w796, write buffer=":*RST;:trig:sour tlin;\n:trig:dir sour;\n:trig:outp sour;\n:TRIG:DEL 0;\n:SYST:AZER:STAT OFF", error in (no error)=w795) -> (VISA resource name out=w813:refnum<visa-resource-name>, error out=w808:errorcluster)  [unwired: 1 out]
                      n105 = VISA Write(VISA resource name=w803, write buffer=":syst:pres;:trac:cle;:trig:del 1;:sens:volt:delt on;\n:sens:volt:nplc 1;\n:trig:del 0.1;:trig:sour ext", error in (no error)=w802) -> (VISA resource name out=w815:refnum<visa-resource-name>, error out=w814:errorcluster)  [unwired: 1 out]
                      n106 = call <instrlib>:"Configure Buffer.vi"("error in (no error)"=w814, "Buffer Source (0: None)"=w818, "Buffer Size (2)"="Size Of Buffer Used For One Measurement", "VISA resource name"=w815) -> ("error out"=w819:errorcluster, "VISA resource name out"=w822:refnum<visa-resource-name>)  [unwired: 6 in]
                      n107 = call <instrlib>:"Configure Output.vi"("Source Mode  (0: Voltage)"=w792, "error in (no error)"=w808, "Compliance  Level (0.1)"=w791, "Output Level (0)"=w790, "VISA resource name"=w813) -> ("error out"=w807:errorcluster, "VISA resource name out"=w789:refnum<visa-resource-name>)  [unwired: 5 in]
                      n108 = Number To Decimal String(number="Size Of Buffer Used For One Measurement") -> (decimal integer string=w809:string)  [unwired: 1 in]
                      n109 = call <instrlib>:"Configure Voltage Parameters.vi"("VISA resource name"=w822, "Measurement (1: Voltage Channel 1)"=w817, "Voltage Resolution (8)"=8, "Range Value (12)"=12.0, "Autorange (T: Enable)"=TRUE, "error in (no error)"=w819) -> ("VISA resource name out"=w821:refnum<visa-resource-name>, "error out"=w820:errorcluster)  [unwired: 8 in]
                      n110 = call <instrlib>:"Configure Measurements.vi"("VISA resource name"=w821, "Measurement (0: Voltage Channel 1)"=w804, "Integration Rate (5)"=5.0, "error in (no error)"=w820) -> ("VISA resource name out"=w806:refnum<visa-resource-name>, "error out"=w805:errorcluster)  [unwired: 10 in]
                      n111 = call <instrlib>:"Enable Buffer Storage.vi"("error in (no error)"=w805, "VISA resource name"=w806) -> ("error out"=w799:errorcluster, "VISA resource name out"=w800:refnum<visa-resource-name>)  [unwired: 8 in]
                      n112 = Concatenate Strings(":TRAC:CLE;:TRAC:FEED SENS;:TRAC:POIN " ("write buffer"), w809, ";:TRIG:COUN " ("write buffer"), w809, ";:TRAC:FEED:CONT NEXT" ("write buffer")) -> (w788:string)
                      n113 = VISA Write(VISA resource name=w789, write buffer=w788, error in (no error)=w807) -> (VISA resource name out=w798:refnum<visa-resource-name>, error out=w797:errorcluster)  [unwired: 1 out]
                    }
                    frame #1 {
                      n114 = VISA Write(VISA resource name=w831, write buffer=":OUTP ON;:init") -> (VISA resource name out=w830:refnum<visa-resource-name>, error out=w829:errorcluster)  [unwired: 1 in, 1 out]
                    }
                    frame #2 {
                      n115 = Wait (ms)(milliseconds to wait=u32 1000) -> ()  [unwired: 1 out]
                    }
                    frame #3 {
                      # "2182"
                      # "2400"
                      n116 = VISA Write(VISA resource name=w851, write buffer=":TRAC:DATA?", error in (no error)=w850) -> (VISA resource name out=w861:refnum<visa-resource-name>, error out=w860:errorcluster)  [unwired: 1 out]
                      n117 = VISA Write(VISA resource name=w849, write buffer=":TRAC:DATA?", error in (no error)=w848) -> (VISA resource name out=w870:refnum<visa-resource-name>, error out=w869:errorcluster)  [unwired: 1 out]
                      n118 = VISA Read(VISA resource name=w861, byte count=u32 100000, error in (no error)=w860) -> (VISA resource name out=w844:refnum<visa-resource-name>, read buffer=w857:string, error out=w843:errorcluster)  [unwired: 1 out]
                      n119 = VISA Read(VISA resource name=w870, byte count=u32 100000, error in (no error)=w869) -> (VISA resource name out=w842:refnum<visa-resource-name>, read buffer=w867:string, error out=w841:errorcluster)  [unwired: 1 out]
                      n120 = call <vilib>:"Delimited String to 1D String Array.vi"("delimiter"=",+" ("delimiter (Tab)"), "delimited string"=w857) -> ("string array"=w853:string[])  [unwired: 9 in]
                      n121 = call <vilib>:"Delimited String to 1D String Array.vi"("delimiter"=",+" ("delimiter (Tab)"), "delimited string"=w867) -> ("string array"=w862:string[])  [unwired: 9 in]
                      n122 = Build Array(0.0 ("array")) -> (w855:dbl[])
                      n123 = Build Array(0.0 ("array")) -> (w865:dbl[])
                      n124 = Delete From Array(array=w855, index=0) -> (array with subset deleted=w845:dbl[])  [unwired: 1 in, 1 out]
                      n125 = Delete From Array(array=w865, index=0) -> (array with subset deleted=w863:dbl[])  [unwired: 1 in, 1 out]
                      n126 = for {
                        N: w840 -> [_]
                        shift-right: [w876] -> w846
                        shift-left: w845 -> [w875]
                        tunnel: w853 -> [w874]
                        i -> [w882]
                        n127 = Multiply(x=w882, y=5) -> (x*y=w881:i32)
                        n128 = Add(x=w881, y=1) -> (x+y=w878:i32)
                        n129 = Index Array(array=w874, index=w878) -> (element=w873:string)
                        n130 = Scan From String(input string=w873) -> (output 1=w877:dbl)  [unwired: 4 in, 3 out]
                        n131 = Build Array (concatenate)(w875, w877) -> (w876:dbl[])
                      }
                      n132 = for {
                        N: w840 -> [_]
                        shift-right: [w885] -> w847
                        shift-left: w863 -> [w884]
                        tunnel: w862 -> [w883] mode=indexing
                        n133 = Scan From String(format string="%f", input string=w883) -> (output 1=w886:dbl)  [unwired: 3 in, 3 out]
                        n134 = Build Array (concatenate)(w884, w886) -> (w885:dbl[])
                      }
                    }
                    frame #4 {
                      n135 = VISA Write(VISA resource name=w894, write buffer=":ABORT;\n:OUTP OFF;\n*RST" ("data"), error in (no error)=w893) -> (VISA resource name out=w888:refnum<visa-resource-name>, error out=w891:errorcluster)  [unwired: 1 out]
                    }
                    frame #5 {
                      n136 = VISA Write(VISA resource name=w898, write buffer=":STAT:PRES;\n:*CLS" ("data"), error in (no error)=w897) -> (VISA resource name out=w895:refnum<visa-resource-name>, error out=w896:errorcluster)  [unwired: 1 out]
                    }
                  }
                  n137 = call-poly <vilib>:"Mean.vi"("X"=w758) -> ("mean"=w782:dbl, "error"=w770:i32)
                  n138 = Number To Engineering String(4:w770) -> (0:w769:string)  [unwired: 3 in]
                  n139 = call-poly <vilib>:"Mean.vi"("X"=w757) -> ("mean"=w781:dbl, "error"=w774:i32)
                  n140 = Divide(x=w782, y=w781) -> (x/y=w780:dbl)
                  n141 = Number To Engineering String(4:w774) -> (0:w773:string)  [unwired: 3 in]
                  n142 = Build Array(w782, w781, w780) -> (w783:dbl[])
                  n143 = Number To Engineering String(4:w781) -> (0:w775:string)  [unwired: 3 in]
                  n144 = Number To Engineering String(4:w780) -> (0:w767:string)  [unwired: 3 in]
                  n145 = Number To Engineering String(4:w782) -> (0:w771:string)  [unwired: 3 in]
                  n146 = Concatenate Strings("Measured Source current: " ("string"), w775, w773, " measured voltage: " ("string"), w771, w769, " calculated resistance: " ("string"), w767) -> (w779:string)
                }
                frame "SR830" {
                }
                frame "SR830 and 6221" {
                }
              }
              n147 = Concatenate Strings(w678, w684, w680) -> (w682:string)
              "Measurement Log" <- w682
              n148 = call "add measurements to map.vi"("Measurement Values"=w676, "Measurement Names"=w677, "Measurements Map in"=w675) -> ("Measurements Map Out"=w673:map{string, dbl[]})  [unwired: 2 in]
              n149 = for {
                tunnel: [w703] -> _ mode=indexing
                tunnel: w673 -> [w703] mode=indexing
                tunnel: [w702] -> w672 mode=indexing
                tunnel: [w701] -> w671 mode=indexing
                n150 = Unbundle(w703) -> (w702:string, "Array"=w701:dbl[])
              }
              "Results Description" <- w672
              n151 = Search and Replace String(replace all?=TRUE, input string=w682, search string=w680) -> (number of replacements=w679:i32)  [unwired: 5 in, 3 out]
              n152 = property on="Measurement Log" class="Str"("Text.Scroll Position"=w679) -> ()  [unwired: 2 in, 2 out]
              n153 = Transpose 2D Array(2D array=w671) -> (transposed array=→"Results":dbl[][])
              n154 = Array Size(array=w672) -> (size(s)=w674:i32)
              n155 = property on="Results" class="Arr (strict)"("Number of Columns"=w674) -> ()  [unwired: 2 in, 2 out]
              n156 = property on="Results Description" class="Arr (strict)"("Number of Columns"=w674) -> ()  [unwired: 2 in, 2 out]
            }
            n157 = VISA Write(VISA resource name=w597, write buffer="ROUT:OPEN:ALL", error in (no error)=w579) -> (VISA resource name out=w596:refnum<visa-resource-name>, error out=w595:errorcluster)  [unwired: 1 out]
            n158 = case shown="\"2400 and  2182\"" w613 {
              tunnel: w612 -> [_ w632 w637 _ _]
              tunnel: w611 -> [w628 w631 w638 _ _]
              tunnel: [w628 w630 w633 _ _] -> w582
              tunnel: w585 -> [_ _ w636 _ _]
              tunnel: w584 -> [w627 w629 w635 _ _]
              tunnel: [w627 w629 w634 _ _] -> w581
              frame "DAQ6510", Default {
              }
              frame "2400 Only" {
                n159 = call <instrlib>:"Close.vi"("error in (no error)"=w631, "VISA resource name"=w632) -> ("error out"=w630:errorcluster)  [unwired: 9 in]
              }
              frame "2400 and  2182" {
                n160 = call <instrlib>:"Close.vi"("error in (no error)"=w638, "VISA resource name"=w637) -> ("error out"=w633:errorcluster)  [unwired: 9 in]
                n161 = call <instrlib>:"Close.vi"("error in (no error)"=w635, "VISA resource name"=w636) -> ("error out"=w634:errorcluster)  [unwired: 9 in]
              }
              frame "SR830" {
              }
              frame "SR830 and 6221" {
              }
            }
            n162 = call <instrlib>:"Close.vi"("error in (no error)"=w595, "VISA resource name"=w596) -> ("error out"=w578:errorcluster)  [unwired: 9 in]
            n163 = call "save measurements.vi"("Save path"=w601, "Measurements In"=w583) -> ()  [unwired: 12 in, 2 out]
            n164 = Build Array(w578, w582, w581) -> (→"Comms Errors":errorcluster[])
          }
        }
        n165 = case shown="\"2400 and  2182\"" "Radio Buttons" {
          tunnel: [w558 w560 w562 w563 w566] -> w551
          tunnel: [w558 w561 w562 w563 w565] -> w550
          tunnel: [TRUE w561 w562 TRUE w566] -> w546
          tunnel: [w558 w561 w562 w563 w566] -> w545
          tunnel: [w558 w560 w562 w563 w565] -> w538
          frame "DAQ6510", Default {
            w558 = FALSE
          }
          frame "2400 Only" {
            w561 = TRUE
            w560 = FALSE
          }
          frame "2400 and  2182" {
            w562 = TRUE
          }
          frame "SR830" {
            w563 = FALSE
          }
          frame "SR830 and 6221" {
            w565 = FALSE
            w566 = TRUE
          }
        }
        n166 = property on="Size Of Buffer Used For One Measurement" class="DigNum (strict)"("Visible"=w538) -> ()  [unwired: 2 in, 2 out]
        n167 = property on="Measurement Repeats" class="DigNum (strict)"("Visible"=w546) -> ()  [unwired: 2 in, 2 out]
        n168 = property on="Current (µA)" class="DigNum (strict)"("Visible"=w550) -> ()  [unwired: 2 in, 2 out]
        n169 = property on="Measure Instrument" class="VISAName"("Visible"=w551) -> ()  [unwired: 2 in, 2 out]
        n170 = property on="Compliance voltage (V)" class="DigNum (strict)"("Visible"=w545) -> ()  [unwired: 2 in, 2 out]
      }
      frame 3 {
        # "Magnetic Op."
      }
      frame 4 {
        # "Calculations"
        # "Save File - saves collected data into a (csv) file and asks for a file path if not already given"
        n171 = Look In Map(map=w916, key="Resistance") -> (value=w914:dbl[])  [unwired: 1 in, 1 out]
        n172 = Build Array("Top Film R est.", "Bottm Film R est.", "RA est.") -> (w924:dbl[])
        n173 = case shown="True" "Fit Data" {
          tunnel: w919 -> [_ w944]
          tunnel: w924 -> [_ w942]
          tunnel: [dbl[] [0.0, 0.0, 0.0] w933] -> w921
          tunnel: w914 -> [_ w931]
          frame False {
          }
          frame True {
            # "Calculated R"
            # "Mean probe spacing"
            n174 = Index Array(array=w944, index (col)=4 ("disabled index (col)")) -> (element=w943:i64[])  [unwired: 1 in]
            n175 = vi-ref "modelFunction.vi"() -> (w941:refnum<vi>)
            n176 = call-poly <vilib>:"Nonlinear Curve Fit.vi"("Y"=w931, "f(x,a)"=w941, "X"=w943, "initial parameters"=w942) -> ("best fit parameters"=w933:dbl[], "error out"=→"error out (fitting model)":errorcluster)  [unwired: 6 in, 4 out]
            n177 = Index Array(array=w933, index=0) -> (element=→"Top Film R":dbl)
            n178 = Index Array(array=w933, index=1) -> (element=→"Bottom Film R":dbl)
            n179 = Index Array(array=w933, index=2) -> (element=→"RA":dbl)
          }
        }
        n180 = case shown="True" "Save File" {
          tunnel: w919 -> [_ w965]
          tunnel: string[] ["I+", "V+", "V-", "I-", "x (mean probe spacing)", "V", "I (µA)", "R (=V/I)"] -> [_ w961]
          tunnel: string[] ["R (t)", "R (b)", "RA"] -> [_ w953]
          tunnel: w921 -> [_ w946]
          tunnel: w917 -> [_ w945]
          frame False {
          }
          frame True {
            n181 = call-poly <vilib>:"Write Delimited Spreadsheet.vi"("file path (dialog if empty)"=w945, "1D data"=w961, "delimiter (\\t)"="," ("delimiter (\\t)")) -> ("new file path (Not A Path if cancelled)"=w963:path, "error out"=w962:errorcluster)  [unwired: 11 in]
            n182 = call-poly <vilib>:"Write Delimited Spreadsheet.vi"("file path (dialog if empty)"=w963, "format (%d)"="%.6f" ("format (%.3f)"), "2D data"=w965, "append to file? (new file:F)"=TRUE, "error in (no error)"=w962, "delimiter (\\t)"="," ("delimiter (\\t)")) -> ("new file path (Not A Path if cancelled)"=w955:path, "error out"=w954:errorcluster)  [unwired: 8 in]
            n183 = call-poly <vilib>:"Write Delimited Spreadsheet.vi"("file path (dialog if empty)"=w955, "format (%s)"="%.6f" ("format (%.3f)"), "1D data"=w953, "append to file? (new file:F)"=TRUE, "error in (no error)"=w954, "delimiter (\\t)"="," ("delimiter (\\t)")) -> ("new file path (Not A Path if cancelled)"=w948:path, "error out"=w947:errorcluster)  [unwired: 8 in]
            n184 = call-poly <vilib>:"Write Delimited Spreadsheet.vi"("file path (dialog if empty)"=w948, "format (%.3f)"="%.6f", "1D data"=w946, "append to file? (new file:F)"=TRUE, "error in (no error)"=w947, "delimiter (\\t)"="," ("delimiter (\\t)")) -> ("error out"=→"error file out":errorcluster)  [unwired: 8 in, 1 out]
          }
        }
        "Measurements Map Out" <- w916
      }
    }
    n185 = case shown="False" "Exit Camera 2" {
      tunnel: ["" "Exit camera"] -> w151
      frame False {
      }
      frame True {
      }
    }
    n186 = case shown="False" "Init Camera 2" {
      tunnel: ["" "Init camera"] -> w154
      frame False {
      }
      frame True {
      }
    }
    n187 = case shown="False" "Init Camera" {
      tunnel: ["" "Init camera"] -> w167
      frame False {
      }
      frame True {
      }
    }
    n188 = case shown="False" "Exit Camera" {
      tunnel: ["" "Exit camera"] -> w164
      frame False {
      }
      frame True {
      }
    }
    n189 = property on="Image first camera" class="Pict"("ZoomFactor"=0.175) -> ()  [unwired: 2 in, 2 out]
    n190 = property on="Image second camera" class="Pict"("ZoomFactor"=0.175) -> ()  [unwired: 2 in, 2 out]
    n191 = Concatenate Strings(w154, w151) -> (w153:string)
    n192 = Concatenate Strings(w167, w164) -> (w166:string)
    n193 = case shown="\"Init camera\"" w153 {
      tunnel: w144 -> [w295 w326 w391]
      tunnel: w143 -> [w296 w325 w390]
      tunnel: [w305 w328 w369] -> w146
      tunnel: [w306 w327 w370] -> w150
      tunnel: [TRUE FALSE FALSE] -> w148
      frame "Exit camera" {
        # "Close .Net Referenz"
        # "Is acquisition running?"
        # "Stop Acquisition"
        # "Close Camera"
        n194 = control-ref of="Init Camera 2"() -> (w290:refnum<vi>)
        n195 = control-ref of="Exit Camera 2"() -> (w289:refnum<vi>)
        n196 = property class="Camera"(reference=w295, error in=w296) -> (error out=w304:errorcluster, "Acquisition"=w303:refnum<k24>)  [unwired: 1 out]
        n197 = property class="Bool"(reference=w290, "Disabled"=u8 0 ("Deaktiviert")) -> ()  [unwired: 1 in, 2 out]
        n198 = property class="Bool"(reference=w289, "Disabled"=u8 2 ("Deaktiviert")) -> ()  [unwired: 1 in, 2 out]
        n199 = invoke class="Acquisition" method="HasStarted"(reference=w303, error in=w304) -> (reference out=w297:refnum<k24>, error out=w300:errorcluster, "bValue"=w302:bool)  [unwired: 2 in, 1 out]
        n200 = invoke class="Acquisition" method="ToString"(reference=w297, error in=w300) -> (error out=w299:errorcluster, "ToString"=w298:string)  [unwired: 1 in, 1 out]
        n201 = call <instrlib>:"Error_Handling.vi"("Error String"=w298, "Error In"=w299) -> ("Error Out"=w301:errorcluster)  [unwired: 9 in]
        n202 = case shown="True" w302 {
          tunnel: [w314 w323] -> w293
          tunnel: w301 -> [w314 w324]
          tunnel: w295 -> [w313 w315]
          tunnel: [w313 w315] -> w294
          frame False {
          }
          frame True {
            n203 = property class="Camera"(reference=w315, error in=w324) -> (error out=w319:errorcluster, "Acquisition"=w320:refnum<k24>)  [unwired: 1 out]
            n204 = invoke class="Acquisition" method="Stop"(reference=w320, error in=w319) -> (reference out=w317:refnum<k24>, error out=w318:errorcluster, "Stop"=w316:i32)  [unwired: 1 in]
            n205 = invoke class="Acquisition" method="ToString"(reference=w317, error in=w318) -> (error out=w322:errorcluster, "ToString"=w321:string)  [unwired: 1 in, 1 out]
            n206 = call <instrlib>:"Error_Handling.vi"("Error Code"=w316, "Error String"=w321, "Error In"=w322) -> ("Error Out"=w323:errorcluster)  [unwired: 8 in]
          }
        }
        n207 = invoke class="Camera" method="Exit"(reference=w294, error in=w293) -> (reference out=w305:refnum<k24>, error out=w309:errorcluster, "Exit"=w308:i32)  [unwired: 1 in]
        n208 = invoke class="Camera" method="ToString"(reference=w305, error in=w309) -> (error out=w310:errorcluster, "ToString"=w311:string)  [unwired: 1 in, 1 out]
        n209 = call <instrlib>:"Error_Handling.vi"("Error Code"=w308, "Error String"=w311, "Error In"=w310) -> ("Error Out"=w307:errorcluster)  [unwired: 8 in]
        n210 = Close Reference ("Close Referenz")(reference=w305, error in (no error)=w307) -> (error out=w306:errorcluster)
      }
      frame Default {
        # "Has acquisition started?"
        # "Show Image"
        n211 = property class="Camera"(reference=w326, error in=w325) -> (error out=w337:errorcluster, "Acquisition"=w336:refnum<k24>)  [unwired: 1 out]
        n212 = invoke class="Acquisition" method="HasStarted"(reference=w336, error in=w337) -> (reference out=w332:refnum<k24>, error out=w331:errorcluster, "HasStarted"=w330:i32, "bValue"=w335:bool)  [unwired: 2 in]
        n213 = invoke class="Acquisition" method="ToString"(reference=w332, error in=w331) -> (error out=w334:errorcluster, "ToString"=w333:string)  [unwired: 1 in, 1 out]
        n214 = call <instrlib>:"Error_Handling.vi"("Error Code"=w330, "Error String"=w333, "Error In"=w334) -> ("Error Out"=w329:errorcluster)  [unwired: 8 in]
        n215 = case shown="False" w335 {
          tunnel: [w340 w346] -> w327
          tunnel: w329 -> [w340 w345]
          tunnel: w326 -> [w339 w341]
          tunnel: [w339 w341] -> w328
          frame False {
          }
          frame True {
            # "Memory"
            n216 = property class="Camera"(reference=w341, error in=w345) -> (error out=w348:errorcluster, "Memory"=w349:refnum<k24>)  [unwired: 1 out]
            n217 = invoke class="Memory" method="GetActive"(reference=w349, error in=w348) -> (reference out=w355:refnum<k24>, error out=w354:errorcluster, "GetActive"=w356:i32, "s32MemId"=w347:i32)  [unwired: 2 in]
            n218 = invoke class="Memory" method="ToString"(reference=w355, error in=w354) -> (error out=w352:errorcluster, "ToString"=w353:string)  [unwired: 1 in, 1 out]
            n219 = call <instrlib>:"Error_Handling.vi"("Error Code"=w356, "Error String"=w353, "Error In"=w352) -> ("Error Out"=w357:errorcluster)  [unwired: 8 in]
            n220 = property class="Camera"(reference=w341, error in=w357) -> (error out=w351:errorcluster, "Memory"=w350:refnum<k24>)  [unwired: 1 out]
            n221 = invoke class="Memory" method="CopyToArray"(reference=w350, error in=w351, "s32MemId"=w347) -> (reference out=w360:refnum<k24>, error out=w361:errorcluster, "CopyToArray"=w362:i32, "u8Image"=w342:u8[])  [unwired: 2 in, 1 out]
            n222 = invoke class="Memory" method="ToString"(reference=w360, error in=w361) -> (error out=w358:errorcluster, "ToString"=w359:string)  [unwired: 1 in, 1 out]
            n223 = call <instrlib>:"Error_Handling.vi"("Error Code"=w362, "Error String"=w359, "Error In"=w358) -> ("Error Out"=w343:errorcluster)  [unwired: 8 in]
            n224 = call <instrlib>:"ArrayToImage.vi"("Error In"=w343, "InArray"=w342, ".NET (Reference)"=w341) -> ("Error Out"=w346:errorcluster, "Image"=→"Image second camera":picture)  [unwired: 7 in]
          }
        }
      }
      frame "Init camera" {
        w371 = 1 items=["IS_DONT_WAIT", "IS_WAIT"] ("Wait")
        w398 = 0 items=["RGB 32"=0, "RGB 24"=1, "Y8 Monochrom"=6] ("Mode")
        # "SubVI Example for \nGetDefault Timing"
        # "SubVI Example for \nMemory allocation"
        # "SubVI Example for \nTiming"
        # "SubVI Example for \nCamera Init"
        # "Pixelformat"
        n225 = control-ref of="Init Camera 2"() -> (w366:refnum<vi>)
        n226 = control-ref of="Exit Camera 2"() -> (w364:refnum<vi>)
        n227 = property class="Bool"(reference=w366, "Disabled"=u8 2 ("Deaktiviert")) -> ()  [unwired: 1 in, 2 out]
        n228 = property class="Bool"(reference=w364, "Disabled"=u8 0 ("Deaktiviert")) -> ()  [unwired: 1 in, 2 out]
        n229 = call <instrlib>:"SubVI_Example_CameraInit.vi"("Error In"=w390, "Camera ID"="Camera ID 3", "Init Camera Flag"=TRUE, ".NET (Reference)"=w391) -> ("Error Out"=w395:errorcluster, ".NET (Reference)"=w369:refnum<k24>)  [unwired: 6 in]
        n230 = property class="Camera"(reference=w369, error in=w395) -> (error out=w396:errorcluster, "PixelFormat"=w397:refnum<k24>)  [unwired: 1 out]
        n231 = invoke class="PixelFormat" method="Set"(reference=w397, error in=w396, "mode"=w398) -> (reference out=w393:refnum<k24>, error out=w387:errorcluster, "Set"=w392:i32)  [unwired: 1 in, 1 out]
        n232 = invoke class="PixelFormat" method="ToString"(reference=w393, error in=w387) -> (error out=w386:errorcluster, "ToString"=w394:string)  [unwired: 1 in, 1 out]
        n233 = call <instrlib>:"Error_Handling.vi"("Error Code"=w392, "Error String"=w394, "Error In"=w386) -> ("Error Out"=w383:errorcluster)  [unwired: 8 in]
        n234 = call <instrlib>:"SubVI_Example_GetDefault_Timing.vi"(".NET (Reference)"=w369, "Error In"=w383) -> ("Pixelclock"=w380:i32, "Exposure time"=w381:dbl, "Framerate"=w382:dbl, "Error Out"=w379:errorcluster)  [unwired: 10 in]
        n235 = call <instrlib>:"SubVI_Example_Timing.vi"(".NET (Reference)"=w369, "Pixelclock"=w380, "Exposure time"=w381, "Framerate"=w382, "Error In"=w379) -> ("Error Out"=w385:errorcluster)  [unwired: 7 in, 3 out]
        n236 = call <instrlib>:"SubVI_Example_MemoryAllocation.vi"(".NET (Reference)"=w369, "Error In"=w385) -> ("Serial Number"=→"Serial Number 2":string, "Error Out"=w368:errorcluster)  [unwired: 13 in, 3 out]
        n237 = property class="Camera"(reference=w369, error in=w368) -> (error out=w377:errorcluster, "Acquisition"=w378:refnum<k24>)  [unwired: 1 out]
        n238 = invoke class="Acquisition" method="Capture"(reference=w378, error in=w377, "param"=w371) -> (reference out=w373:refnum<k24>, error out=w374:errorcluster, "Capture"=w372:i32)  [unwired: 1 in, 1 out]
        n239 = invoke class="Acquisition" method="ToString"(reference=w373, error in=w374) -> (error out=w376:errorcluster, "ToString"=w375:string)  [unwired: 1 in, 1 out]
        n240 = call <instrlib>:"Error_Handling.vi"("Error Code"=w372, "Error String"=w375, "Error In"=w376) -> ("Error Out"=w370:errorcluster)  [unwired: 8 in]
      }
    }
    n241 = case shown="Default" w166 {
      tunnel: w157 -> [w409 w440 w505]
      tunnel: w156 -> [w410 w439 w504]
      tunnel: [w419 w442 w484] -> w159
      tunnel: [w420 w441 w485] -> w163
      tunnel: [TRUE FALSE FALSE] -> w161
      frame "Exit camera" {
        # "Close .Net Referenz"
        # "Is acquisition running?"
        # "Stop Acquisition"
        # "Close Camera"
        n242 = control-ref of="Init Camera"() -> (w404:refnum<vi>)
        n243 = control-ref of="Exit Camera"() -> (w403:refnum<vi>)
        n244 = property class="Camera"(reference=w409, error in=w410) -> (error out=w418:errorcluster, "Acquisition"=w417:refnum<k24>)  [unwired: 1 out]
        n245 = property class="Bool"(reference=w404, "Disabled"=u8 0 ("Deaktiviert")) -> ()  [unwired: 1 in, 2 out]
        n246 = property class="Bool"(reference=w403, "Disabled"=u8 2 ("Deaktiviert")) -> ()  [unwired: 1 in, 2 out]
        n247 = invoke class="Acquisition" method="HasStarted"(reference=w417, error in=w418) -> (reference out=w411:refnum<k24>, error out=w414:errorcluster, "bValue"=w416:bool)  [unwired: 2 in, 1 out]
        n248 = invoke class="Acquisition" method="ToString"(reference=w411, error in=w414) -> (error out=w413:errorcluster, "ToString"=w412:string)  [unwired: 1 in, 1 out]
        n249 = call <instrlib>:"Error_Handling.vi"("Error String"=w412, "Error In"=w413) -> ("Error Out"=w415:errorcluster)  [unwired: 9 in]
        n250 = case shown="True" w416 {
          tunnel: [w428 w437] -> w407
          tunnel: w415 -> [w428 w438]
          tunnel: w409 -> [w427 w429]
          tunnel: [w427 w429] -> w408
          frame False {
          }
          frame True {
            n251 = property class="Camera"(reference=w429, error in=w438) -> (error out=w433:errorcluster, "Acquisition"=w434:refnum<k24>)  [unwired: 1 out]
            n252 = invoke class="Acquisition" method="Stop"(reference=w434, error in=w433) -> (reference out=w431:refnum<k24>, error out=w432:errorcluster, "Stop"=w430:i32)  [unwired: 1 in]
            n253 = invoke class="Acquisition" method="ToString"(reference=w431, error in=w432) -> (error out=w436:errorcluster, "ToString"=w435:string)  [unwired: 1 in, 1 out]
            n254 = call <instrlib>:"Error_Handling.vi"("Error Code"=w430, "Error String"=w435, "Error In"=w436) -> ("Error Out"=w437:errorcluster)  [unwired: 8 in]
          }
        }
        n255 = invoke class="Camera" method="Exit"(reference=w408, error in=w407) -> (reference out=w419:refnum<k24>, error out=w423:errorcluster, "Exit"=w422:i32)  [unwired: 1 in]
        n256 = invoke class="Camera" method="ToString"(reference=w419, error in=w423) -> (error out=w424:errorcluster, "ToString"=w425:string)  [unwired: 1 in, 1 out]
        n257 = call <instrlib>:"Error_Handling.vi"("Error Code"=w422, "Error String"=w425, "Error In"=w424) -> ("Error Out"=w421:errorcluster)  [unwired: 8 in]
        n258 = Close Reference ("Close Referenz")(reference=w419, error in (no error)=w421) -> (error out=w420:errorcluster)
      }
      frame Default {
        # "Has acquisition started?"
        n259 = property class="Camera"(reference=w440, error in=w439) -> (error out=w451:errorcluster, "Acquisition"=w450:refnum<k24>)  [unwired: 1 out]
        n260 = invoke class="Acquisition" method="HasStarted"(reference=w450, error in=w451) -> (reference out=w446:refnum<k24>, error out=w445:errorcluster, "HasStarted"=w444:i32, "bValue"=w449:bool)  [unwired: 2 in]
        n261 = invoke class="Acquisition" method="ToString"(reference=w446, error in=w445) -> (error out=w448:errorcluster, "ToString"=w447:string)  [unwired: 1 in, 1 out]
        n262 = call <instrlib>:"Error_Handling.vi"("Error Code"=w444, "Error String"=w447, "Error In"=w448) -> ("Error Out"=w443:errorcluster)  [unwired: 8 in]
        n263 = case shown="True" w449 {
          tunnel: [w454 w460] -> w441
          tunnel: w443 -> [w454 w459]
          tunnel: w440 -> [w453 w457]
          tunnel: [w453 w457] -> w442
          frame False {
            # "Show Image"
          }
          frame True {
            # "Memory"
            n264 = property class="Camera"(reference=w457, error in=w459) -> (error out=w462:errorcluster, "Memory"=w463:refnum<k24>)  [unwired: 1 out]
            n265 = invoke class="Memory" method="GetActive"(reference=w463, error in=w462) -> (reference out=w469:refnum<k24>, error out=w468:errorcluster, "GetActive"=w470:i32, "s32MemId"=w461:i32)  [unwired: 2 in]
            n266 = invoke class="Memory" method="ToString"(reference=w469, error in=w468) -> (error out=w466:errorcluster, "ToString"=w467:string)  [unwired: 1 in, 1 out]
            n267 = call <instrlib>:"Error_Handling.vi"("Error Code"=w470, "Error String"=w467, "Error In"=w466) -> ("Error Out"=w471:errorcluster)  [unwired: 8 in]
            n268 = property class="Camera"(reference=w457, error in=w471) -> (error out=w465:errorcluster, "Memory"=w464:refnum<k24>)  [unwired: 1 out]
            n269 = invoke class="Memory" method="CopyToArray"(reference=w464, error in=w465, "s32MemId"=w461) -> (reference out=w474:refnum<k24>, error out=w475:errorcluster, "CopyToArray"=w476:i32, "u8Image"=w456:u8[])  [unwired: 2 in, 1 out]
            n270 = invoke class="Memory" method="ToString"(reference=w474, error in=w475) -> (error out=w472:errorcluster, "ToString"=w473:string)  [unwired: 1 in, 1 out]
            n271 = call <instrlib>:"Error_Handling.vi"("Error Code"=w476, "Error String"=w473, "Error In"=w472) -> ("Error Out"=w458:errorcluster)  [unwired: 8 in]
            n272 = call <instrlib>:"ArrayToImage.vi"("Error In"=w458, "InArray"=w456, ".NET (Reference)"=w457) -> ("Error Out"=w460:errorcluster, "Image"=→"Image first camera":picture)  [unwired: 7 in]
          }
        }
      }
      frame "Init camera" {
        w486 = 1 items=["IS_DONT_WAIT", "IS_WAIT"] ("Wait")
        w512 = 0 items=["RGB 32"=0, "RGB 24"=1, "Y8 Monochrom"=6] ("Mode")
        # "SubVI Example for \nGetDefault Timing"
        # "SubVI Example for \nMemory allocation"
        # "SubVI Example for \nTiming"
        # "SubVI Example for \nCamera Init"
        # "Pixelformat"
        n273 = control-ref of="Init Camera"() -> (w480:refnum<vi>)
        n274 = control-ref of="Exit Camera"() -> (w478:refnum<vi>)
        n275 = call <instrlib>:"SubVI_Example_CameraInit.vi"("Error In"=w504, "Camera ID"="Camera ID 1", "Init Camera Flag"=TRUE, ".NET (Reference)"=w505) -> ("Error Out"=w509:errorcluster, ".NET (Reference)"=w484:refnum<k24>)  [unwired: 6 in]
        n276 = property class="Bool"(reference=w480, "Disabled"=u8 2 ("Deaktiviert")) -> ()  [unwired: 1 in, 2 out]
        n277 = property class="Bool"(reference=w478, "Disabled"=u8 0 ("Deaktiviert")) -> ()  [unwired: 1 in, 2 out]
        n278 = property class="Camera"(reference=w484, error in=w509) -> (error out=w510:errorcluster, "PixelFormat"=w511:refnum<k24>)  [unwired: 1 out]
        n279 = invoke class="PixelFormat" method="Set"(reference=w511, error in=w510, "mode"=w512) -> (reference out=w507:refnum<k24>, error out=w501:errorcluster, "Set"=w506:i32)  [unwired: 1 in, 1 out]
        n280 = invoke class="PixelFormat" method="ToString"(reference=w507, error in=w501) -> (error out=w500:errorcluster, "ToString"=w508:string)  [unwired: 1 in, 1 out]
        n281 = call <instrlib>:"Error_Handling.vi"("Error Code"=w506, "Error String"=w508, "Error In"=w500) -> ("Error Out"=w497:errorcluster)  [unwired: 8 in]
        n282 = call <instrlib>:"SubVI_Example_GetDefault_Timing.vi"(".NET (Reference)"=w484, "Error In"=w497) -> ("Pixelclock"=w494:i32, "Exposure time"=w495:dbl, "Framerate"=w496:dbl, "Error Out"=w482:errorcluster)  [unwired: 10 in]
        n283 = call <instrlib>:"SubVI_Example_Timing.vi"(".NET (Reference)"=w484, "Pixelclock"=w494, "Exposure time"=w495, "Framerate"=w496, "Error In"=w482) -> ("Error Out"=w499:errorcluster)  [unwired: 7 in, 3 out]
        n284 = call <instrlib>:"SubVI_Example_MemoryAllocation.vi"(".NET (Reference)"=w484, "Error In"=w499) -> ("Serial Number"=→"Serial Number 1":string, "Error Out"=w483:errorcluster)  [unwired: 13 in, 3 out]
        n285 = property class="Camera"(reference=w484, error in=w483) -> (error out=w492:errorcluster, "Acquisition"=w493:refnum<k24>)  [unwired: 1 out]
        n286 = invoke class="Acquisition" method="Capture"(reference=w493, error in=w492, "param"=w486) -> (reference out=w488:refnum<k24>, error out=w489:errorcluster, "Capture"=w487:i32)  [unwired: 1 in, 1 out]
        n287 = invoke class="Acquisition" method="ToString"(reference=w488, error in=w489) -> (error out=w491:errorcluster, "ToString"=w490:string)  [unwired: 1 in, 1 out]
        n288 = call <instrlib>:"Error_Handling.vi"("Error Code"=w487, "Error String"=w490, "Error In"=w491) -> ("Error Out"=w485:errorcluster)  [unwired: 8 in]
      }
    }
    n289 = case shown="False" "steps /\n continuous \ntoggle" {
      tunnel: w130 -> [w187 w263]
      tunnel: w129 -> [w186 w262]
      tunnel: [w205 w269] -> w128
      tunnel: [w178 w275] -> w118
      tunnel: "up a1" -> [w204 w271]
      tunnel: "down a1" -> [w202 w270]
      tunnel: "up all" -> [w185 w258]
      tunnel: "down all" -> [w184 w259]
      tunnel: "down a3" -> [w192 w267]
      tunnel: "up a3" -> [w193 w266]
      tunnel: "down a2" -> [w190 w261]
      tunnel: "up a2" -> [w191 w260]
      tunnel: w123 -> [_ w273]
      tunnel: [_ w274] -> w127
      tunnel: [_ w254] -> w126
      tunnel: w122 -> [_ w251]
      tunnel: [_ w252] -> w124
      tunnel: w120 -> [_ w249]
      tunnel: [_ w253] -> w125
      tunnel: w121 -> [_ w250]
      frame False {
        n290 = flat-sequence {
          tunnel: w187 -> [w220]
          tunnel: w186 -> [w223]
          tunnel: w193 -> [w218]
          tunnel: "a3" ("Combo Box") -> [w216]
          tunnel: "Step size" -> [w219]
          tunnel: w192 -> [w217]
          tunnel: [w222] -> w196
          tunnel: [w221] -> w195
          tunnel: [w225] -> _
          tunnel: [w226] -> w180
          tunnel: w196 -> [w226]
          tunnel: w195 -> [w225]
          frame #0 {
            n291 = call "Picomotor step single.vi"("Step size"=w219, "Combo Box"=w216, "error in (no error)"=w223, "down a1"=w217, "up a1"=w218, "VISA Refnum in"=w220) -> ("error out"=w222:errorcluster, "VISA Refnum out"=w221:refnum<visa-resource-name>)  [unwired: 4 in]
          }
          frame #1 {
            n292 = Wait (ms)(milliseconds to wait=u32 100) -> ()  [unwired: 1 out]
          }
        }
        n293 = flat-sequence {
          tunnel: w187 -> [w242]
          tunnel: w186 -> [w245]
          tunnel: w204 -> [w240]
          tunnel: "a1" ("Combo Box") -> [w238]
          tunnel: "Step size" -> [w241]
          tunnel: w202 -> [w239]
          tunnel: [w244] -> w201
          tunnel: [w243] -> w200
          tunnel: [w247] -> w205
          tunnel: [w248] -> w182
          tunnel: w201 -> [w248]
          tunnel: w200 -> [w247]
          frame #0 {
            n294 = call "Picomotor step single.vi"("Step size"=w241, "Combo Box"=w238, "error in (no error)"=w245, "down a1"=w239, "up a1"=w240, "VISA Refnum in"=w242) -> ("error out"=w244:errorcluster, "VISA Refnum out"=w243:refnum<visa-resource-name>)  [unwired: 4 in]
          }
          frame #1 {
            n295 = Wait (ms)(milliseconds to wait=u32 100) -> ()  [unwired: 1 out]
          }
        }
        n296 = flat-sequence {
          tunnel: w187 -> [w231]
          tunnel: w186 -> [w234]
          tunnel: w191 -> [w229]
          tunnel: "a2" ("Combo Box") -> [w227]
          tunnel: "Step size" -> [w230]
          tunnel: w190 -> [w228]
          tunnel: [w233] -> w199
          tunnel: [w232] -> w198
          tunnel: [w236] -> _
          tunnel: [w237] -> w181
          tunnel: w199 -> [w237]
          tunnel: w198 -> [w236]
          frame #0 {
            n297 = call "Picomotor step single.vi"("Step size"=w230, "Combo Box"=w227, "error in (no error)"=w234, "down a1"=w228, "up a1"=w229, "VISA Refnum in"=w231) -> ("error out"=w233:errorcluster, "VISA Refnum out"=w232:refnum<visa-resource-name>)  [unwired: 4 in]
          }
          frame #1 {
            n298 = Wait (ms)(milliseconds to wait=u32 100) -> ()  [unwired: 1 out]
          }
        }
        n299 = flat-sequence {
          tunnel: [w212] -> w189
          tunnel: [w211] -> w188
          tunnel: w187 -> [w210]
          tunnel: w186 -> [w209]
          tunnel: w185 -> [w208]
          tunnel: w184 -> [w207]
          tunnel: "Step size" -> [w206]
          tunnel: [w214] -> _
          tunnel: [w215] -> w179
          tunnel: w189 -> [w215]
          tunnel: w188 -> [w214]
          frame #0 {
            n300 = call "Picomotor step multi.vi"("Step size"=w206, "error in (no error)"=w209, "down a1"=w207, "up a1"=w208, "VISA Refnum in"=w210) -> ("error out"=w212:errorcluster, "VISA Refnum out"=w211:refnum<visa-resource-name>)  [unwired: 5 in]
          }
          frame #1 {
            n301 = Wait (ms)(milliseconds to wait=u32 100) -> ()  [unwired: 1 out]
          }
        }
        n302 = Merge Errors(w182, w181, w180, w179) -> (w178:errorcluster)
      }
      frame True {
        n303 = call "Picomotor single motor continuous.vi"("Enum"=w273, "Combo Box"="a1", "error in (no error)"=w262, "down"=w270, "up"=w271, "VISA Refnum in"=w263) -> ("error out"=w268:errorcluster, "Numeric"=w274:i32, "VISA Refnum out"=w269:refnum<visa-resource-name>)  [unwired: 3 in]
        n304 = call "Picomotor single motor continuous.vi"("Enum"=w250, "Combo Box"="a3", "error in (no error)"=w262, "down"=w267, "up"=w266, "VISA Refnum in"=w263) -> ("error out"=w256:errorcluster, "Numeric"=w253:i32)  [unwired: 3 in, 1 out]
        n305 = call "Picomotor single motor continuous.vi"("Enum"=w251, "Combo Box"="a2", "error in (no error)"=w262, "down"=w261, "up"=w260, "VISA Refnum in"=w263) -> ("error out"=w257:errorcluster, "Numeric"=w254:i32)  [unwired: 3 in, 1 out]
        n306 = call "Picomotor all motors continuous.vi"("Enum"=w249, "error in (no error)"=w262, "down"=w259, "up"=w258, "VISA Refnum in"=w263) -> ("error out"=w255:errorcluster, "Numeric"=w252:i32)  [unwired: 4 in, 1 out]
        n307 = Merge Errors(w268, w257, w256, w255) -> (w275:errorcluster)
      }
    }
    n308 = call <instrlib>:"SubVI_Example_SyncEventLoop.vi"("Error In"=w150, "use sync"=w148, ".NET (Reference)"=w146) -> ("Error Out"=w145:errorcluster, "Synchronize (ms)"=w149:dbl)  [unwired: 7 in]
    "Error Camera 2" <- w145
    n309 = call <instrlib>:"SubVI_Example_SyncEventLoop.vi"("Error In"=w163, "use sync"=w161, ".NET (Reference)"=w159) -> ("Error Out"=w158:errorcluster, "Synchronize (ms)"=w162:dbl)  [unwired: 7 in]
    "Error Camera 1" <- w158
    n310 = Wait Until Next ms Multiple(millisecond multiple=w162) -> ()  [unwired: 1 out]
    n311 = Wait Until Next ms Multiple(millisecond multiple=w149) -> ()  [unwired: 1 out]
    n312 = case shown="False" "stop" {
      tunnel: w128 -> [w278 w283]
      tunnel: w118 -> [w277 w282]
      tunnel: [w278 w281] -> w117
      tunnel: [w277 w280] -> w119
      tunnel: [w276 w279] -> w141
      tunnel: "stop" -> [w276 w279]
      frame False {
      }
      frame True {
        n313 = call "Picomotor Write.vi"("error in (no error)"=w282, "String 3"="sto", "VISA Refnum in"=w283) -> ("error out"=w280:errorcluster, "VISA Refnum out"=w281:refnum<visa-resource-name>)  [unwired: 6 in, 1 out]
      }
    }
    n314 = Merge Errors(w119, w118) -> (w142:errorcluster)
  }
  n315 = VISA Close(VISA resource name=w1, error in (no error)=w2) -> (error out=→"error":errorcluster)
